vi "函数类型2测试.vi"() -> ()   [LabVIEW 2010]
uses:
  全局量/试验配置信息.vi
panel:
  out "starttest":bool
  in  "记录跳变次数":i32
  in  "变化量":dbl
  in  "当前波动值":dbl
  in  "最近一次跳变防线值":i32
  out "bRecv":bool
  out "bSend":bool
  in  "发送值状态":i32
  in  "反馈值":i32
  in  "发送值":dbl
  out "合格？":bool[][](array[boolean])
  in  "btn_反选":bool
  in  "btn_全选":bool
  out "退出？":bool
  in  "数组_选择":bool[](array[boolean])
  in  "第几组数据":i32
  in  "A_32":bool
  in  "A_31":bool
  in  "A_30":bool
  in  "A_29":bool
  in  "A_28":bool
  in  "A_27":bool
  in  "A_26":bool
  in  "A_25":bool
  in  "A_24":bool
  in  "A_23":bool
  in  "A_22":bool
  in  "A_21":bool
  in  "A_20":bool
  in  "A_19":bool
  in  "A_18":bool
  in  "A_17":bool
  in  "A_16":bool
  in  "A_15":bool
  in  "A_14":bool
  in  "A_13":bool
  in  "A_12":bool
  in  "A_11":bool
  in  "A_10":bool
  in  "A_9":bool
  in  "A_8":bool
  in  "A_7":bool
  in  "A_6":bool
  in  "A_5":bool
  in  "A_4":bool
  in  "A_3":bool
  in  "A_2":bool
  in  "A_1":bool
  in  "btn_取消":bool
  in  "btn_开始测试":bool
  out "light_32":bool
  out "light_31":bool
  out "light_30":bool
  out "light_29":bool
  out "light_28":bool
  out "light_27":bool
  out "light_26":bool
  out "light_25":bool
  out "light_24":bool
  out "light_23":bool
  out "light_22":bool
  out "light_21":bool
  out "light_20":bool
  out "light_19":bool
  out "light_18":bool
  out "light_17":bool
  out "light_16":bool
  out "light_15":bool
  out "light_14":bool
  out "light_13":bool
  out "light_12":bool
  out "light_11":bool
  out "light_10":bool
  out "light_9":bool
  out "light_8":bool
  out "light_7":bool
  out "light_6":bool
  out "light_5":bool
  out "light_4":bool
  out "light_3":bool
  out "light_2":bool
  out "light_1":bool
  in  "跳变值 2":dbl[](array[numeric])
  in  "跳变值 1":dbl[](array[numeric])
  out "Analog_back":string[][](table) caption="表格"
  in  "Analog_IN":string[][](table) caption="表格"
  # "反馈电平状态"
  # "模拟量输入值（V）"
  # "SEND_RISE = 1,//递增\n\tSEND_SUB = 2,//递减\n\tSEND_OVER = 3//发送完毕"
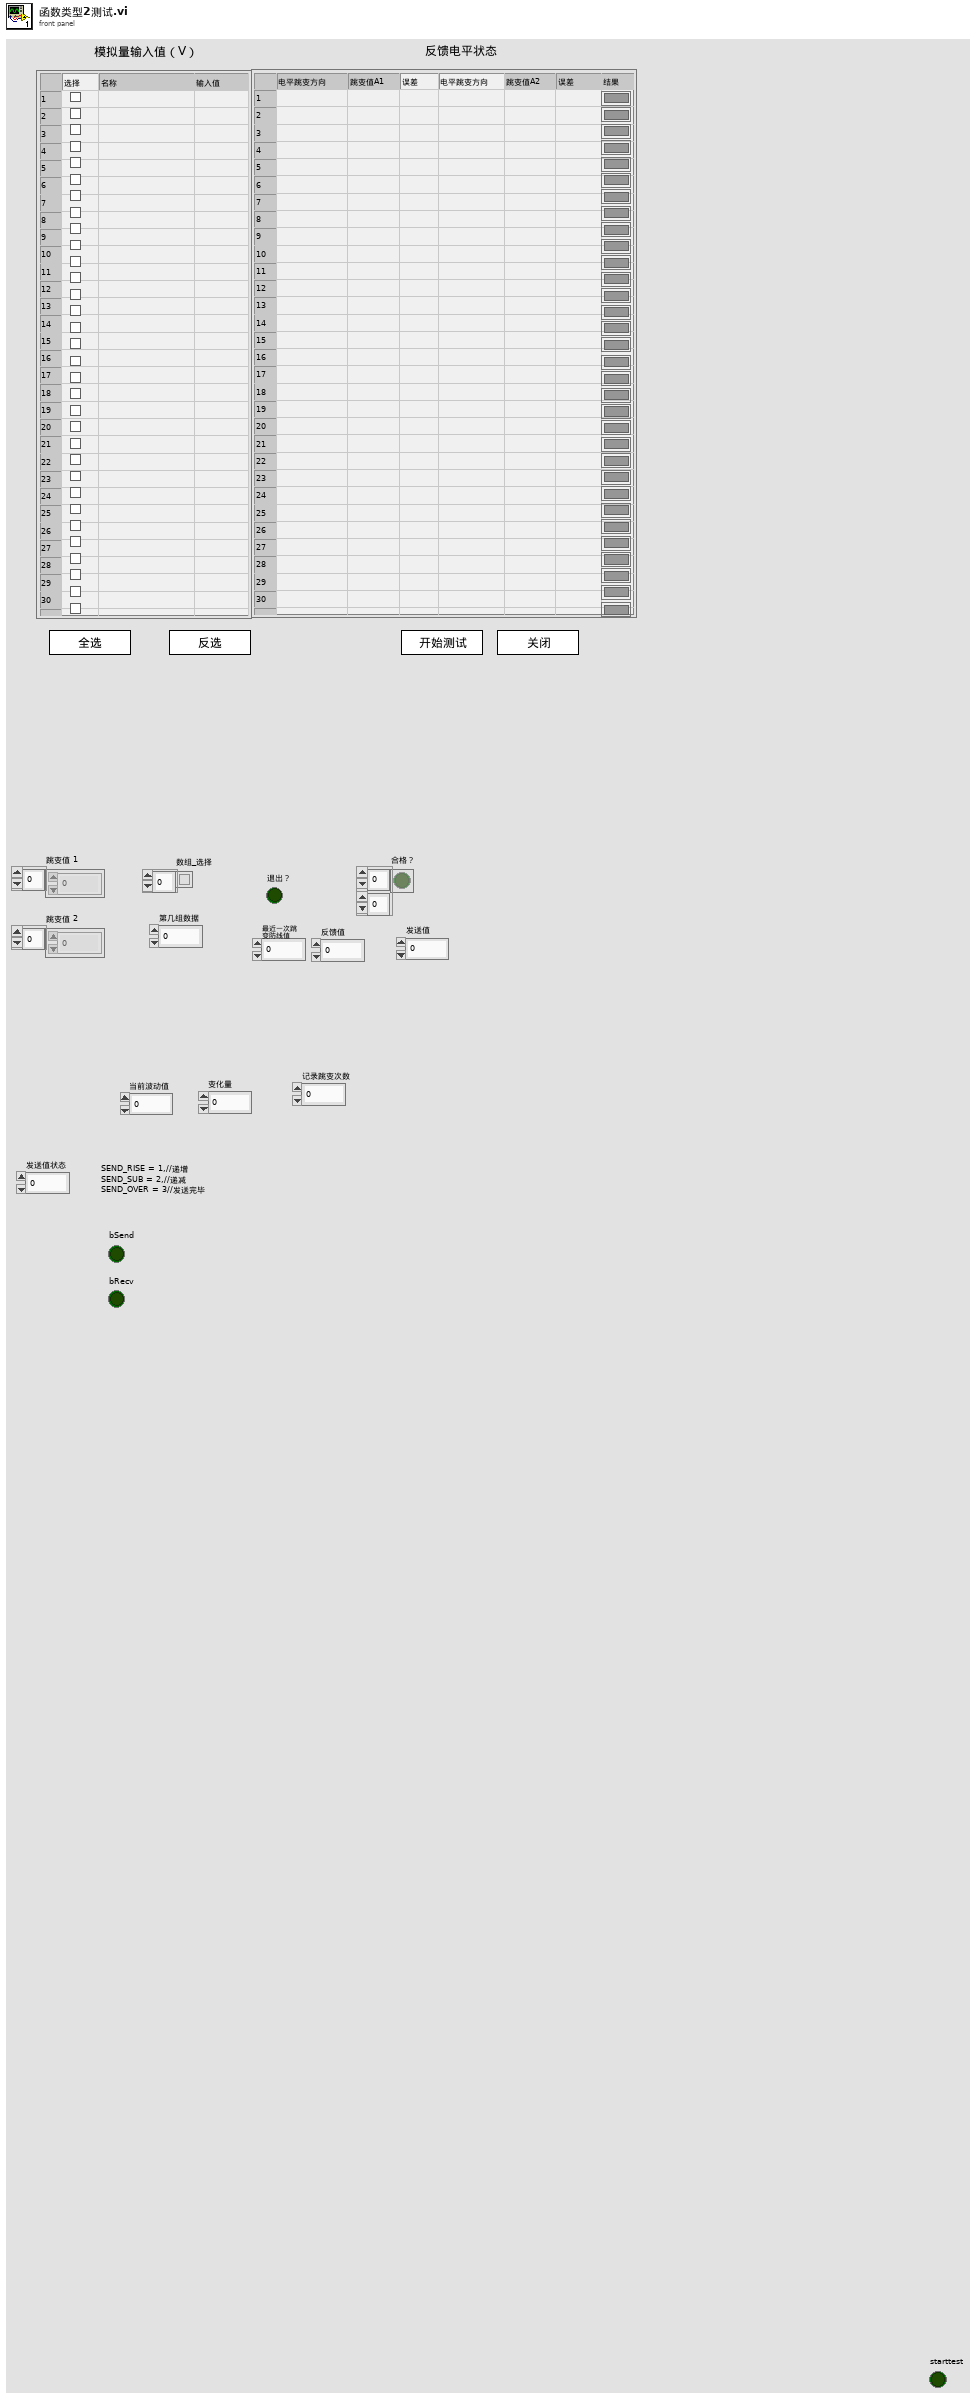
[diagram p1: front panel]
types:
  T1 = enum8{"Enabled", "Disabled", "Disabled and Grayed Out"}
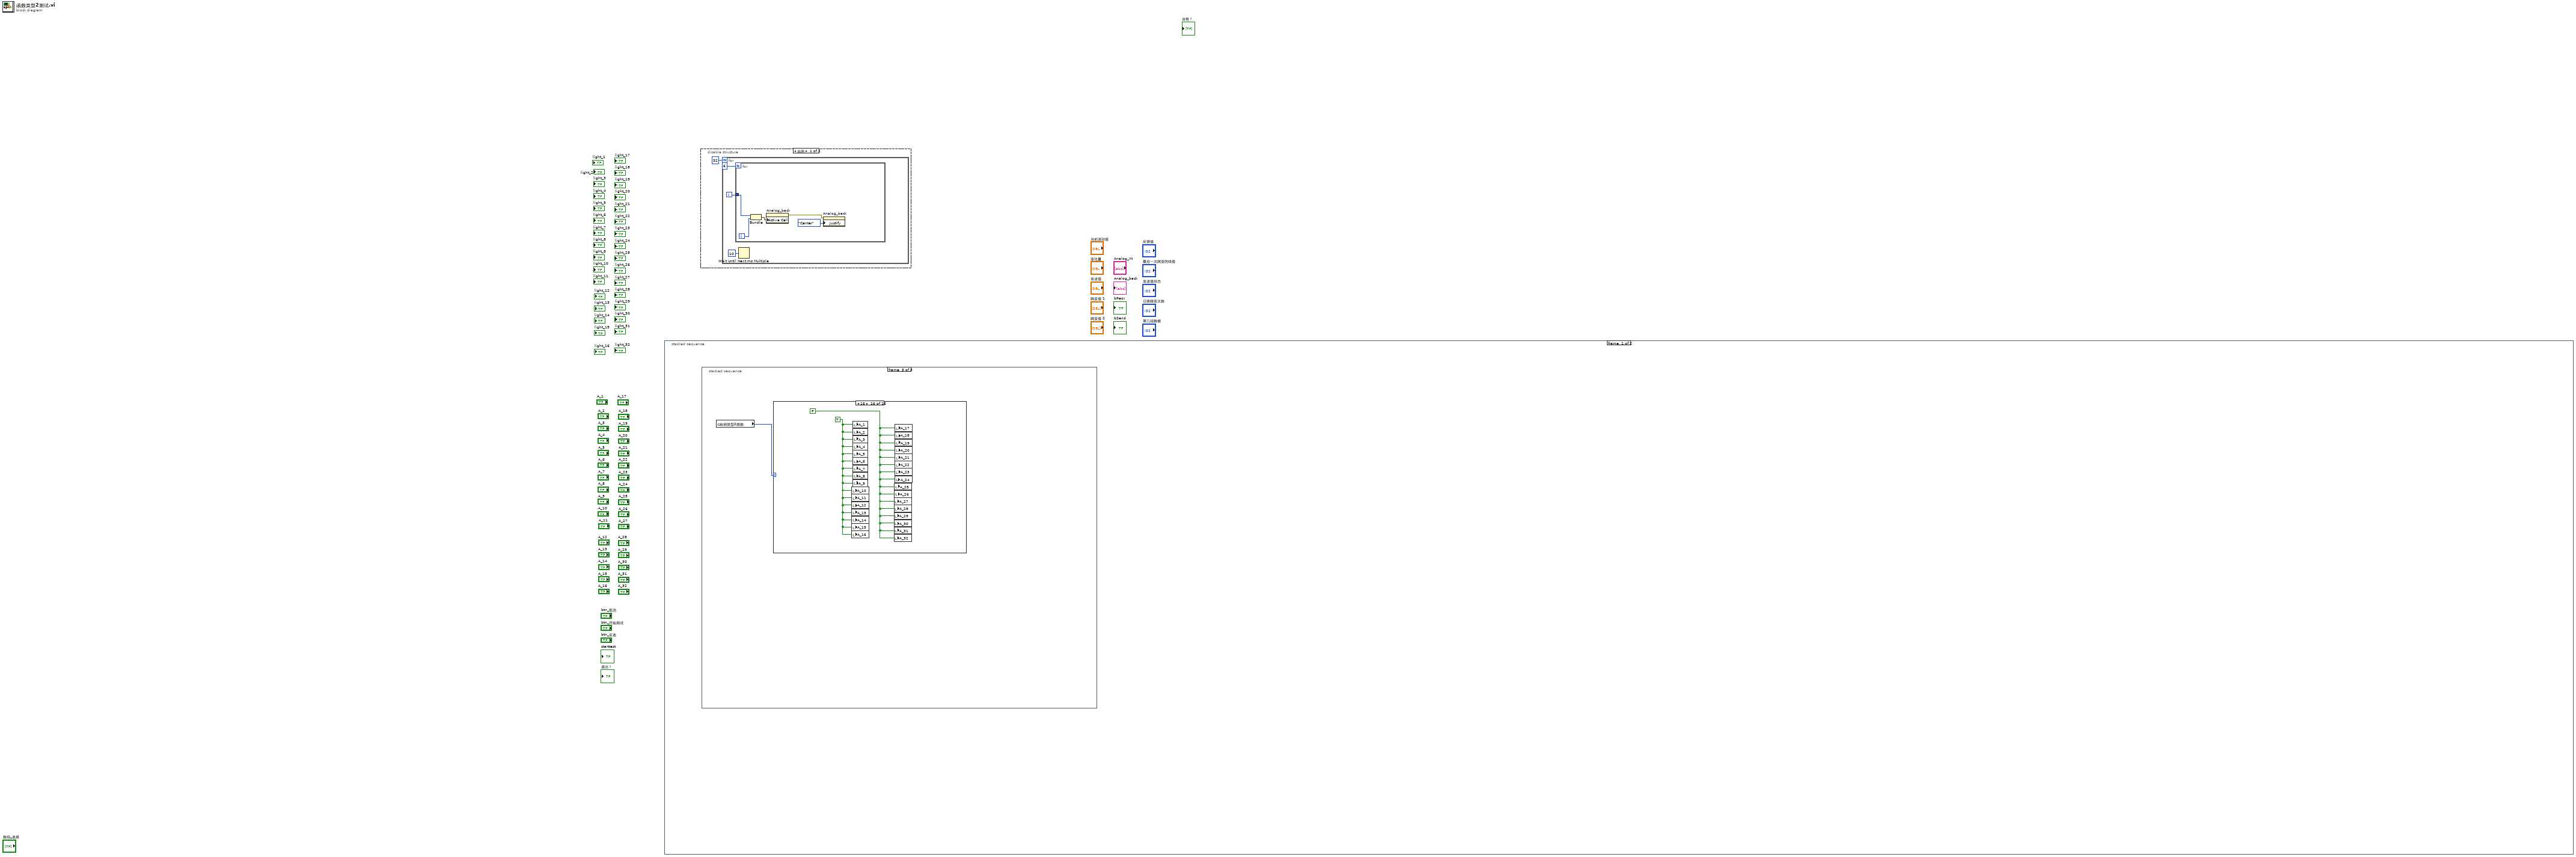
[diagram p0: block diagram]
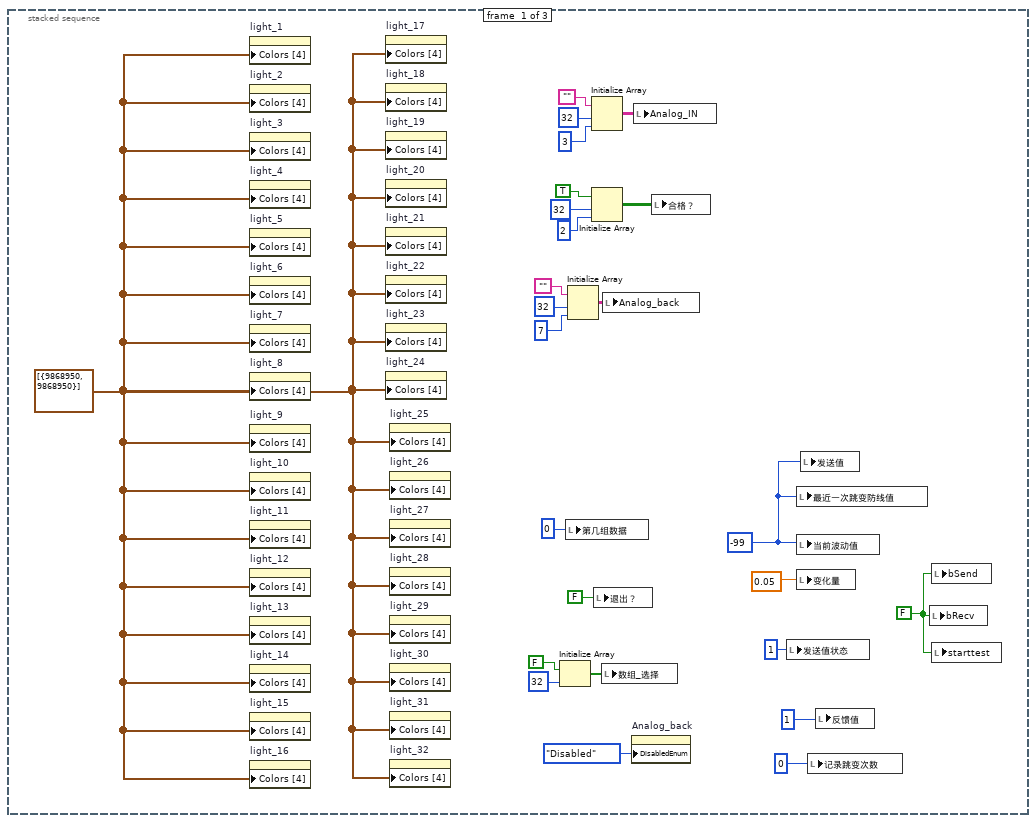
[diagram p3: hidden frame]
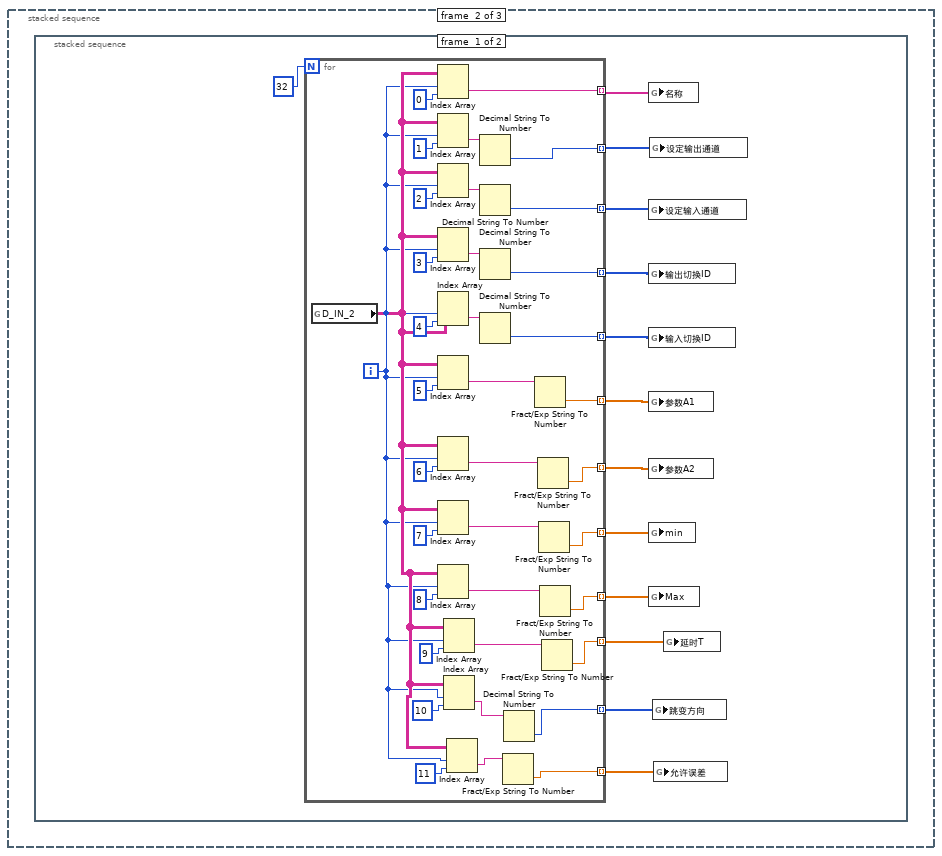
[diagram p4: hidden frame]
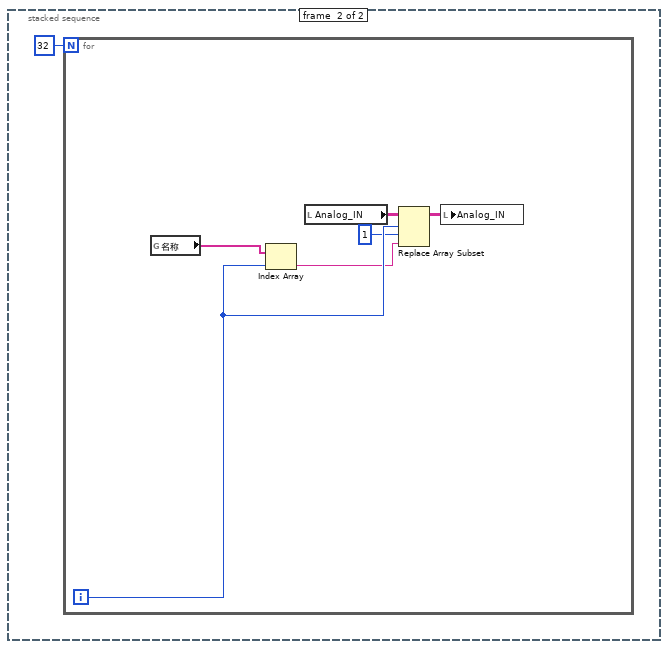
[diagram p5: hidden frame]
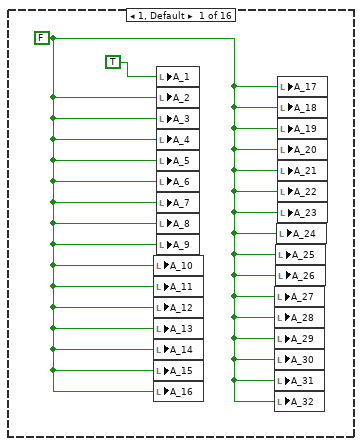
[diagram p6: hidden frame]
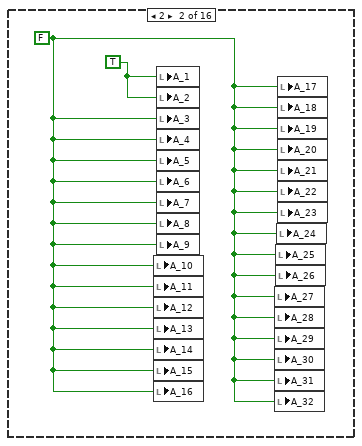
[diagram p7: hidden frame]
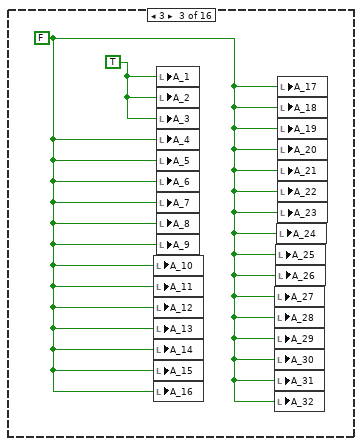
[diagram p8: hidden frame]
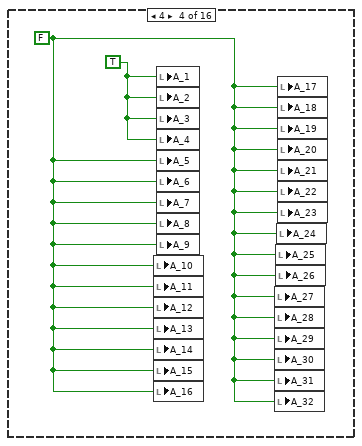
[diagram p9: hidden frame]
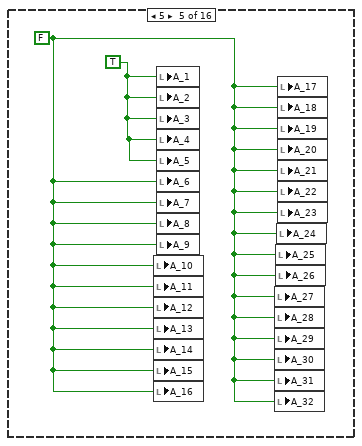
[diagram p10: hidden frame]
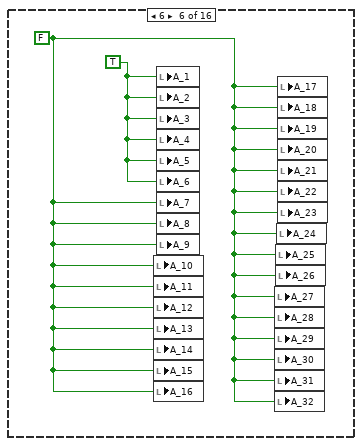
[diagram p11: hidden frame]
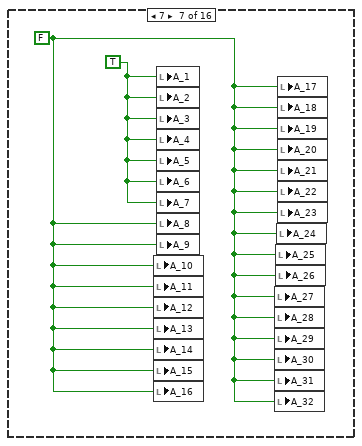
[diagram p12: hidden frame]
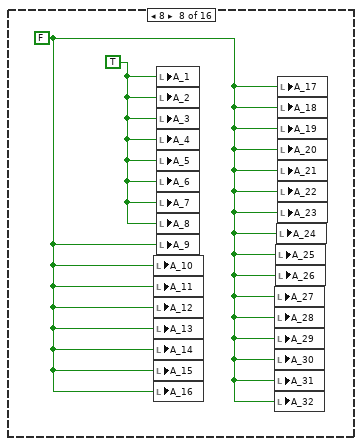
[diagram p13: hidden frame]
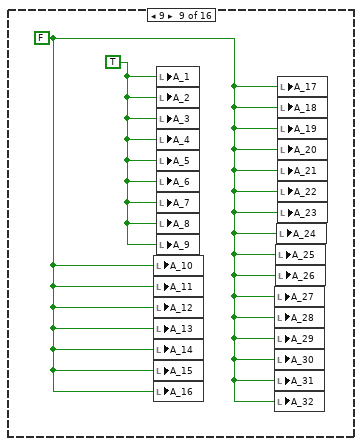
[diagram p14: hidden frame]
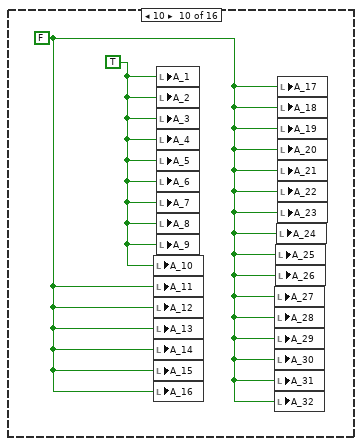
[diagram p15: hidden frame]
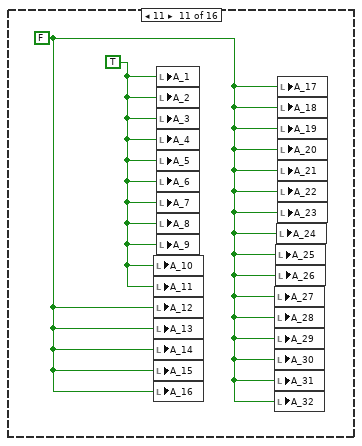
[diagram p16: hidden frame]
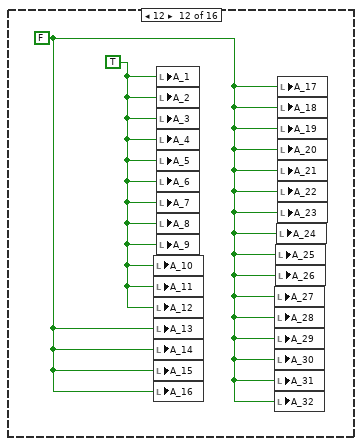
[diagram p17: hidden frame]
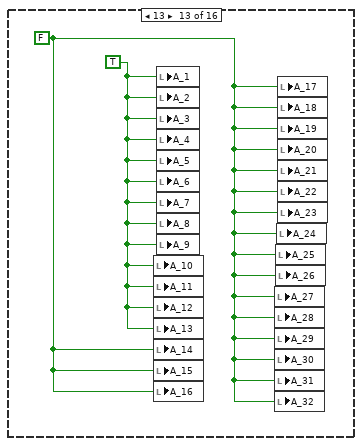
[diagram p18: hidden frame]
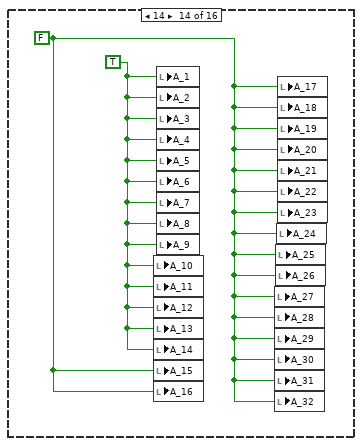
[diagram p19: hidden frame]
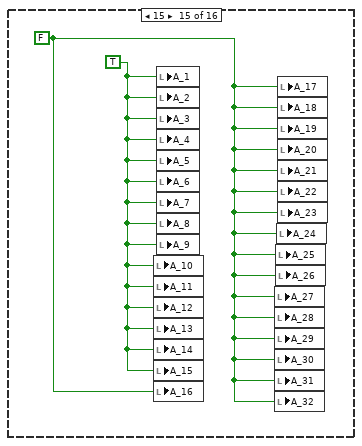
[diagram p20: hidden frame]
diagram:
  n1 = stacked-sequence {
    frame #0 {
      n2 = stacked-sequence {
        frame #0 {
          w9 = -99
          w6 = FALSE
          w21 = cluster{u32, u32}[] [{9868950, 9868950}]
          n3 = property on="light_1" class="Bool (严格)"("Colors [4]"=w21) -> ()  [unwired: 2 in, 2 out]
          n4 = property on="light_2" class="Bool (严格)"("Colors [4]"=w21) -> ()  [unwired: 2 in, 2 out]
          n5 = property on="light_3" class="Bool (严格)"("Colors [4]"=w21) -> ()  [unwired: 2 in, 2 out]
          n6 = property on="light_4" class="Bool (严格)"("Colors [4]"=w21) -> ()  [unwired: 2 in, 2 out]
          n7 = property on="light_5" class="Bool (严格)"("Colors [4]"=w21) -> ()  [unwired: 2 in, 2 out]
          n8 = property on="light_6" class="Bool (严格)"("Colors [4]"=w21) -> ()  [unwired: 2 in, 2 out]
          n9 = property on="light_7" class="Bool (严格)"("Colors [4]"=w21) -> ()  [unwired: 2 in, 2 out]
          n10 = property on="light_8" class="Bool (严格)"("Colors [4]"=w21) -> ()  [unwired: 2 in, 2 out]
          n11 = property on="light_9" class="Bool (严格)"("Colors [4]"=w21) -> ()  [unwired: 2 in, 2 out]
          n12 = property on="light_10" class="Bool (严格)"("Colors [4]"=w21) -> ()  [unwired: 2 in, 2 out]
          n13 = property on="light_11" class="Bool (严格)"("Colors [4]"=w21) -> ()  [unwired: 2 in, 2 out]
          n14 = property on="light_12" class="Bool (严格)"("Colors [4]"=w21) -> ()  [unwired: 2 in, 2 out]
          n15 = property on="light_13" class="Bool (严格)"("Colors [4]"=w21) -> ()  [unwired: 2 in, 2 out]
          n16 = property on="light_14" class="Bool (严格)"("Colors [4]"=w21) -> ()  [unwired: 2 in, 2 out]
          n17 = property on="light_15" class="Bool (严格)"("Colors [4]"=w21) -> ()  [unwired: 2 in, 2 out]
          n18 = property on="light_16" class="Bool (严格)"("Colors [4]"=w21) -> ()  [unwired: 2 in, 2 out]
          n19 = property on="light_17" class="Bool (严格)"("Colors [4]"=w21) -> ()  [unwired: 2 in, 2 out]
          n20 = property on="light_18" class="Bool (严格)"("Colors [4]"=w21) -> ()  [unwired: 2 in, 2 out]
          n21 = property on="light_19" class="Bool (严格)"("Colors [4]"=w21) -> ()  [unwired: 2 in, 2 out]
          n22 = property on="light_20" class="Bool (严格)"("Colors [4]"=w21) -> ()  [unwired: 2 in, 2 out]
          n23 = property on="light_21" class="Bool (严格)"("Colors [4]"=w21) -> ()  [unwired: 2 in, 2 out]
          n24 = property on="light_22" class="Bool (严格)"("Colors [4]"=w21) -> ()  [unwired: 2 in, 2 out]
          n25 = property on="light_23" class="Bool (严格)"("Colors [4]"=w21) -> ()  [unwired: 2 in, 2 out]
          n26 = property on="light_24" class="Bool (严格)"("Colors [4]"=w21) -> ()  [unwired: 2 in, 2 out]
          n27 = property on="light_25" class="Bool (严格)"("Colors [4]"=w21) -> ()  [unwired: 2 in, 2 out]
          n28 = property on="light_26" class="Bool (严格)"("Colors [4]"=w21) -> ()  [unwired: 2 in, 2 out]
          n29 = property on="light_27" class="Bool (严格)"("Colors [4]"=w21) -> ()  [unwired: 2 in, 2 out]
          n30 = property on="light_28" class="Bool (严格)"("Colors [4]"=w21) -> ()  [unwired: 2 in, 2 out]
          n31 = property on="light_29" class="Bool (严格)"("Colors [4]"=w21) -> ()  [unwired: 2 in, 2 out]
          n32 = property on="light_30" class="Bool (严格)"("Colors [4]"=w21) -> ()  [unwired: 2 in, 2 out]
          n33 = property on="light_31" class="Bool (严格)"("Colors [4]"=w21) -> ()  [unwired: 2 in, 2 out]
          n34 = property on="light_32" class="Bool (严格)"("Colors [4]"=w21) -> ()  [unwired: 2 in, 2 out]
          n35 = Initialize Array(FALSE, 32 ("维数大小")) -> (w19:bool[])
          n36 = local write "第几组数据"(0 ("第几组数据")) -> ()
          n37 = Initialize Array("", 32 ("维数大小"), 7 ("维数大小")) -> (w5:string[][])
          n38 = Initialize Array("", 32 ("维数大小"), 3 ("维数大小")) -> (w22:string[][])
          n39 = Initialize Array(TRUE, 32 ("维数大小"), 2 ("维数大小")) -> (w14:bool[][])
          n40 = local write "退出？"(FALSE ("退出？")) -> ()
          n41 = local write "数组_选择"(w19) -> ()
          n42 = local write "Analog_back"(w5) -> ()
          n43 = property on="Analog_back" class="Tbl (严格)"("DisabledEnum"=T1."Disabled" ("禁用")) -> ()  [unwired: 2 in, 2 out]
          n44 = local write "Analog_IN"(w22) -> ()
          n45 = local write "合格？"(w14) -> ()
          n46 = local write "发送值状态"(1 ("发送值状态")) -> ()
          n47 = local write "最近一次跳变防线值"(w9) -> ()
          n48 = local write "当前波动值"(w9) -> ()
          n49 = local write "变化量"(0.05) -> ()
          n50 = local write "发送值"(w9) -> ()
          n51 = local write "记录跳变次数"(0) -> ()
          n52 = local write "反馈值"(1) -> ()
          n53 = local write "bRecv"(w6) -> ()
          n54 = local write "bSend"(w6) -> ()
          n55 = local write "starttest"(w6) -> ()
        }
        frame #1 {
          n56 = stacked-sequence {
            frame #0 {
              n57 = for {
                N: 32 ("维数大小") -> [_]
                tunnel: [w74] -> w32 mode=indexing
                tunnel: [w70] -> w31 mode=indexing
                tunnel: [w68] -> w30 mode=indexing
                tunnel: [w65] -> w29 mode=indexing
                tunnel: [w62] -> w28 mode=indexing
                tunnel: [w59] -> w34 mode=indexing
                tunnel: [w56] -> w35 mode=indexing
                tunnel: [w53] -> w36 mode=indexing
                tunnel: [w50] -> w37 mode=indexing
                tunnel: [w47] -> w38 mode=indexing
                tunnel: [w40] -> w27 mode=indexing
                tunnel: [w39] -> w26 mode=indexing
                i -> [w41]
                n58 = global read "试验配置信息.vi" "D_IN_2"() -> (w42:string[][])
                n59 = Index Array(array=w42, index (row)=w41, index (col)=0 ("禁用的索引 (列)")) -> (element=w74:string)
                n60 = Index Array(array=w42, index (row)=w41, index (col)=1 ("禁用的索引 (列)")) -> (element=w67:string)
                n61 = Index Array(array=w42, index (row)=w41, index (col)=2 ("禁用的索引 (列)")) -> (element=w64:string)
                n62 = Index Array(array=w42, index (row)=w41, index (col)=3 ("禁用的索引 (列)")) -> (element=w60:string)
                n63 = Index Array(array=w42, index (row)=w41, index (col)=4 ("禁用的索引 (列)")) -> (element=w58:string)
                n64 = Index Array(array=w42, index (row)=w41, index (col)=5 ("禁用的索引 (列)")) -> (element=w55:string)
                n65 = Index Array(array=w42, index (row)=w41, index (col)=6 ("禁用的索引 (列)")) -> (element=w51:string)
                n66 = Index Array(array=w42, index (row)=w41, index (col)=7 ("禁用的索引 (列)")) -> (element=w71:string)
                n67 = Index Array(array=w42, index (row)=w41, index (col)=8 ("禁用的索引 (列)")) -> (element=w69:string)
                n68 = Index Array(array=w42, index (row)=w41, index (col)=9 ("禁用的索引 (列)")) -> (element=w48:string)
                n69 = Index Array(array=w42, index (row)=w41, index (col)=10 ("禁用的索引 (列)")) -> (element=w43:string)
                n70 = Index Array(array=w42, index (row)=w41, index (col)=11 ("禁用的索引 (列)")) -> (element=w44:string)
                n71 = Decimal String To Number(string=w67) -> (number=w65:i32)  [unwired: 2 in, 1 out]
                n72 = Decimal String To Number(string=w64) -> (number=w62:i32)  [unwired: 2 in, 1 out]
                n73 = Decimal String To Number(string=w60) -> (number=w59:i32)  [unwired: 2 in, 1 out]
                n74 = Decimal String To Number(string=w58) -> (number=w56:i32)  [unwired: 2 in, 1 out]
                n75 = Fract/Exp String To Number(string=w44) -> (number=w39:dbl)  [unwired: 3 in, 1 out]
                n76 = Decimal String To Number(string=w43) -> (number=w40:i32)  [unwired: 2 in, 1 out]
                n77 = Fract/Exp String To Number(string=w55) -> (number=w53:dbl)  [unwired: 3 in, 1 out]
                n78 = Fract/Exp String To Number(string=w51) -> (number=w50:dbl)  [unwired: 3 in, 1 out]
                n79 = Fract/Exp String To Number(string=w71) -> (number=w70:dbl)  [unwired: 3 in, 1 out]
                n80 = Fract/Exp String To Number(string=w69) -> (number=w68:dbl)  [unwired: 3 in, 1 out]
                n81 = Fract/Exp String To Number(string=w48) -> (number=w47:dbl)  [unwired: 3 in, 1 out]
              }
              n82 = global write "试验配置信息.vi" "名称"(w32) -> ()
              n83 = global write "试验配置信息.vi" "设定输入通道"(w28) -> ()
              n84 = global write "试验配置信息.vi" "输出切换ID"(w34) -> ()
              n85 = global write "试验配置信息.vi" "输入切换ID"(w35) -> ()
              n86 = global write "试验配置信息.vi" "参数A1"(w36) -> ()
              n87 = global write "试验配置信息.vi" "参数A2"(w37) -> ()
              n88 = global write "试验配置信息.vi" "min"(w31) -> ()
              n89 = global write "试验配置信息.vi" "Max"(w30) -> ()
              n90 = global write "试验配置信息.vi" "设定输出通道"(w29) -> ()
              n91 = global write "试验配置信息.vi" "跳变方向"(w27) -> ()
              n92 = global write "试验配置信息.vi" "允许误差"(w26) -> ()
              n93 = global write "试验配置信息.vi" "延时T"(w38) -> ()
            }
            frame #1 {
              n94 = for {
                N: 32 -> [_]
                i -> [w79]
                n95 = global read "试验配置信息.vi" "名称"() -> (w82:string[])
                n96 = Index Array(array=w82, index=w79) -> (element=w78:string)
                n97 = local read "Analog_IN"() -> (w81:string[][])
                n98 = Replace Array Subset(array=w81, new element=w78, index (row)=w79, index (col)=1 ("禁用的索引 (列)")) -> (w80:string[][])
                n99 = local write "Analog_IN"(w80) -> ()
              }
            }
          }
        }
        frame #2 {
          n100 = global read "试验配置信息.vi" "自测类型2路数"() -> (w83:i32)
          n101 = case shown="16" w83 {
            frame 1, Default {
              w85 = FALSE
              n102 = local write "A_10"(w85) -> ()
              n103 = local write "A_11"(w85) -> ()
              n104 = local write "A_12"(w85) -> ()
              n105 = local write "A_13"(w85) -> ()
              n106 = local write "A_14"(w85) -> ()
              n107 = local write "A_15"(w85) -> ()
              n108 = local write "A_16"(w85) -> ()
              n109 = local write "A_1"(TRUE) -> ()
              n110 = local write "A_2"(w85) -> ()
              n111 = local write "A_3"(w85) -> ()
              n112 = local write "A_4"(w85) -> ()
              n113 = local write "A_5"(w85) -> ()
              n114 = local write "A_6"(w85) -> ()
              n115 = local write "A_7"(w85) -> ()
              n116 = local write "A_8"(w85) -> ()
              n117 = local write "A_9"(w85) -> ()
              n118 = local write "A_27"(w85) -> ()
              n119 = local write "A_28"(w85) -> ()
              n120 = local write "A_29"(w85) -> ()
              n121 = local write "A_30"(w85) -> ()
              n122 = local write "A_31"(w85) -> ()
              n123 = local write "A_32"(w85) -> ()
              n124 = local write "A_25"(w85) -> ()
              n125 = local write "A_26"(w85) -> ()
              n126 = local write "A_24"(w85) -> ()
              n127 = local write "A_17"(w85) -> ()
              n128 = local write "A_18"(w85) -> ()
              n129 = local write "A_19"(w85) -> ()
              n130 = local write "A_20"(w85) -> ()
              n131 = local write "A_21"(w85) -> ()
              n132 = local write "A_22"(w85) -> ()
              n133 = local write "A_23"(w85) -> ()
            }
            frame 2 {
              w86 = TRUE
              w87 = FALSE
              n134 = local write "A_10"(w87) -> ()
              n135 = local write "A_11"(w87) -> ()
              n136 = local write "A_12"(w87) -> ()
              n137 = local write "A_13"(w87) -> ()
              n138 = local write "A_14"(w87) -> ()
              n139 = local write "A_15"(w87) -> ()
              n140 = local write "A_16"(w87) -> ()
              n141 = local write "A_1"(w86) -> ()
              n142 = local write "A_2"(w86) -> ()
              n143 = local write "A_3"(w87) -> ()
              n144 = local write "A_4"(w87) -> ()
              n145 = local write "A_5"(w87) -> ()
              n146 = local write "A_6"(w87) -> ()
              n147 = local write "A_7"(w87) -> ()
              n148 = local write "A_8"(w87) -> ()
              n149 = local write "A_9"(w87) -> ()
              n150 = local write "A_27"(w87) -> ()
              n151 = local write "A_28"(w87) -> ()
              n152 = local write "A_29"(w87) -> ()
              n153 = local write "A_30"(w87) -> ()
              n154 = local write "A_31"(w87) -> ()
              n155 = local write "A_32"(w87) -> ()
              n156 = local write "A_25"(w87) -> ()
              n157 = local write "A_26"(w87) -> ()
              n158 = local write "A_24"(w87) -> ()
              n159 = local write "A_17"(w87) -> ()
              n160 = local write "A_18"(w87) -> ()
              n161 = local write "A_19"(w87) -> ()
              n162 = local write "A_20"(w87) -> ()
              n163 = local write "A_21"(w87) -> ()
              n164 = local write "A_22"(w87) -> ()
              n165 = local write "A_23"(w87) -> ()
            }
            frame 3 {
              w88 = TRUE
              w89 = FALSE
              n166 = local write "A_10"(w89) -> ()
              n167 = local write "A_11"(w89) -> ()
              n168 = local write "A_12"(w89) -> ()
              n169 = local write "A_13"(w89) -> ()
              n170 = local write "A_14"(w89) -> ()
              n171 = local write "A_15"(w89) -> ()
              n172 = local write "A_16"(w89) -> ()
              n173 = local write "A_1"(w88) -> ()
              n174 = local write "A_2"(w88) -> ()
              n175 = local write "A_3"(w88) -> ()
              n176 = local write "A_4"(w89) -> ()
              n177 = local write "A_5"(w89) -> ()
              n178 = local write "A_6"(w89) -> ()
              n179 = local write "A_7"(w89) -> ()
              n180 = local write "A_8"(w89) -> ()
              n181 = local write "A_9"(w89) -> ()
              n182 = local write "A_27"(w89) -> ()
              n183 = local write "A_28"(w89) -> ()
              n184 = local write "A_29"(w89) -> ()
              n185 = local write "A_30"(w89) -> ()
              n186 = local write "A_31"(w89) -> ()
              n187 = local write "A_32"(w89) -> ()
              n188 = local write "A_25"(w89) -> ()
              n189 = local write "A_26"(w89) -> ()
              n190 = local write "A_24"(w89) -> ()
              n191 = local write "A_17"(w89) -> ()
              n192 = local write "A_18"(w89) -> ()
              n193 = local write "A_19"(w89) -> ()
              n194 = local write "A_20"(w89) -> ()
              n195 = local write "A_21"(w89) -> ()
              n196 = local write "A_22"(w89) -> ()
              n197 = local write "A_23"(w89) -> ()
            }
            frame 4 {
              w90 = TRUE
              w91 = FALSE
              n198 = local write "A_10"(w91) -> ()
              n199 = local write "A_11"(w91) -> ()
              n200 = local write "A_12"(w91) -> ()
              n201 = local write "A_13"(w91) -> ()
              n202 = local write "A_14"(w91) -> ()
              n203 = local write "A_15"(w91) -> ()
              n204 = local write "A_16"(w91) -> ()
              n205 = local write "A_1"(w90) -> ()
              n206 = local write "A_2"(w90) -> ()
              n207 = local write "A_3"(w90) -> ()
              n208 = local write "A_4"(w90) -> ()
              n209 = local write "A_5"(w91) -> ()
              n210 = local write "A_6"(w91) -> ()
              n211 = local write "A_7"(w91) -> ()
              n212 = local write "A_8"(w91) -> ()
              n213 = local write "A_9"(w91) -> ()
              n214 = local write "A_27"(w91) -> ()
              n215 = local write "A_28"(w91) -> ()
              n216 = local write "A_29"(w91) -> ()
              n217 = local write "A_30"(w91) -> ()
              n218 = local write "A_31"(w91) -> ()
              n219 = local write "A_32"(w91) -> ()
              n220 = local write "A_25"(w91) -> ()
              n221 = local write "A_26"(w91) -> ()
              n222 = local write "A_24"(w91) -> ()
              n223 = local write "A_17"(w91) -> ()
              n224 = local write "A_18"(w91) -> ()
              n225 = local write "A_19"(w91) -> ()
              n226 = local write "A_20"(w91) -> ()
              n227 = local write "A_21"(w91) -> ()
              n228 = local write "A_22"(w91) -> ()
              n229 = local write "A_23"(w91) -> ()
            }
            frame 5 {
              w92 = TRUE
              w93 = FALSE
              n230 = local write "A_10"(w93) -> ()
              n231 = local write "A_11"(w93) -> ()
              n232 = local write "A_12"(w93) -> ()
              n233 = local write "A_13"(w93) -> ()
              n234 = local write "A_14"(w93) -> ()
              n235 = local write "A_15"(w93) -> ()
              n236 = local write "A_16"(w93) -> ()
              n237 = local write "A_1"(w92) -> ()
              n238 = local write "A_2"(w92) -> ()
              n239 = local write "A_3"(w92) -> ()
              n240 = local write "A_4"(w92) -> ()
              n241 = local write "A_5"(w92) -> ()
              n242 = local write "A_6"(w93) -> ()
              n243 = local write "A_7"(w93) -> ()
              n244 = local write "A_8"(w93) -> ()
              n245 = local write "A_9"(w93) -> ()
              n246 = local write "A_27"(w93) -> ()
              n247 = local write "A_28"(w93) -> ()
              n248 = local write "A_29"(w93) -> ()
              n249 = local write "A_30"(w93) -> ()
              n250 = local write "A_31"(w93) -> ()
              n251 = local write "A_32"(w93) -> ()
              n252 = local write "A_25"(w93) -> ()
              n253 = local write "A_26"(w93) -> ()
              n254 = local write "A_24"(w93) -> ()
              n255 = local write "A_17"(w93) -> ()
              n256 = local write "A_18"(w93) -> ()
              n257 = local write "A_19"(w93) -> ()
              n258 = local write "A_20"(w93) -> ()
              n259 = local write "A_21"(w93) -> ()
              n260 = local write "A_22"(w93) -> ()
              n261 = local write "A_23"(w93) -> ()
            }
            frame 6 {
              w94 = TRUE
              w95 = FALSE
              n262 = local write "A_10"(w95) -> ()
              n263 = local write "A_11"(w95) -> ()
              n264 = local write "A_12"(w95) -> ()
              n265 = local write "A_13"(w95) -> ()
              n266 = local write "A_14"(w95) -> ()
              n267 = local write "A_15"(w95) -> ()
              n268 = local write "A_16"(w95) -> ()
              n269 = local write "A_1"(w94) -> ()
              n270 = local write "A_2"(w94) -> ()
              n271 = local write "A_3"(w94) -> ()
              n272 = local write "A_4"(w94) -> ()
              n273 = local write "A_5"(w94) -> ()
              n274 = local write "A_6"(w94) -> ()
              n275 = local write "A_7"(w95) -> ()
              n276 = local write "A_8"(w95) -> ()
              n277 = local write "A_9"(w95) -> ()
              n278 = local write "A_27"(w95) -> ()
              n279 = local write "A_28"(w95) -> ()
              n280 = local write "A_29"(w95) -> ()
              n281 = local write "A_30"(w95) -> ()
              n282 = local write "A_31"(w95) -> ()
              n283 = local write "A_32"(w95) -> ()
              n284 = local write "A_25"(w95) -> ()
              n285 = local write "A_26"(w95) -> ()
              n286 = local write "A_24"(w95) -> ()
              n287 = local write "A_17"(w95) -> ()
              n288 = local write "A_18"(w95) -> ()
              n289 = local write "A_19"(w95) -> ()
              n290 = local write "A_20"(w95) -> ()
              n291 = local write "A_21"(w95) -> ()
              n292 = local write "A_22"(w95) -> ()
              n293 = local write "A_23"(w95) -> ()
            }
            frame 7 {
              w96 = TRUE
              w97 = FALSE
              n294 = local write "A_10"(w97) -> ()
              n295 = local write "A_11"(w97) -> ()
              n296 = local write "A_12"(w97) -> ()
              n297 = local write "A_13"(w97) -> ()
              n298 = local write "A_14"(w97) -> ()
              n299 = local write "A_15"(w97) -> ()
              n300 = local write "A_16"(w97) -> ()
              n301 = local write "A_1"(w96) -> ()
              n302 = local write "A_2"(w96) -> ()
              n303 = local write "A_3"(w96) -> ()
              n304 = local write "A_4"(w96) -> ()
              n305 = local write "A_5"(w96) -> ()
              n306 = local write "A_6"(w96) -> ()
              n307 = local write "A_7"(w96) -> ()
              n308 = local write "A_8"(w97) -> ()
              n309 = local write "A_9"(w97) -> ()
              n310 = local write "A_27"(w97) -> ()
              n311 = local write "A_28"(w97) -> ()
              n312 = local write "A_29"(w97) -> ()
              n313 = local write "A_30"(w97) -> ()
              n314 = local write "A_31"(w97) -> ()
              n315 = local write "A_32"(w97) -> ()
              n316 = local write "A_25"(w97) -> ()
              n317 = local write "A_26"(w97) -> ()
              n318 = local write "A_24"(w97) -> ()
              n319 = local write "A_17"(w97) -> ()
              n320 = local write "A_18"(w97) -> ()
              n321 = local write "A_19"(w97) -> ()
              n322 = local write "A_20"(w97) -> ()
              n323 = local write "A_21"(w97) -> ()
              n324 = local write "A_22"(w97) -> ()
              n325 = local write "A_23"(w97) -> ()
            }
            frame 8 {
              w98 = TRUE
              w99 = FALSE
              n326 = local write "A_10"(w99) -> ()
              n327 = local write "A_11"(w99) -> ()
              n328 = local write "A_12"(w99) -> ()
              n329 = local write "A_13"(w99) -> ()
              n330 = local write "A_14"(w99) -> ()
              n331 = local write "A_15"(w99) -> ()
              n332 = local write "A_16"(w99) -> ()
              n333 = local write "A_1"(w98) -> ()
              n334 = local write "A_2"(w98) -> ()
              n335 = local write "A_3"(w98) -> ()
              n336 = local write "A_4"(w98) -> ()
              n337 = local write "A_5"(w98) -> ()
              n338 = local write "A_6"(w98) -> ()
              n339 = local write "A_7"(w98) -> ()
              n340 = local write "A_8"(w98) -> ()
              n341 = local write "A_9"(w99) -> ()
              n342 = local write "A_27"(w99) -> ()
              n343 = local write "A_28"(w99) -> ()
              n344 = local write "A_29"(w99) -> ()
              n345 = local write "A_30"(w99) -> ()
              n346 = local write "A_31"(w99) -> ()
              n347 = local write "A_32"(w99) -> ()
              n348 = local write "A_25"(w99) -> ()
              n349 = local write "A_26"(w99) -> ()
              n350 = local write "A_24"(w99) -> ()
              n351 = local write "A_17"(w99) -> ()
              n352 = local write "A_18"(w99) -> ()
              n353 = local write "A_19"(w99) -> ()
              n354 = local write "A_20"(w99) -> ()
              n355 = local write "A_21"(w99) -> ()
              n356 = local write "A_22"(w99) -> ()
              n357 = local write "A_23"(w99) -> ()
            }
            frame 9 {
              w100 = TRUE
              w101 = FALSE
              n358 = local write "A_10"(w101) -> ()
              n359 = local write "A_11"(w101) -> ()
              n360 = local write "A_12"(w101) -> ()
              n361 = local write "A_13"(w101) -> ()
              n362 = local write "A_14"(w101) -> ()
              n363 = local write "A_15"(w101) -> ()
              n364 = local write "A_16"(w101) -> ()
              n365 = local write "A_1"(w100) -> ()
              n366 = local write "A_2"(w100) -> ()
              n367 = local write "A_3"(w100) -> ()
              n368 = local write "A_4"(w100) -> ()
              n369 = local write "A_5"(w100) -> ()
              n370 = local write "A_6"(w100) -> ()
              n371 = local write "A_7"(w100) -> ()
              n372 = local write "A_8"(w100) -> ()
              n373 = local write "A_9"(w100) -> ()
              n374 = local write "A_27"(w101) -> ()
              n375 = local write "A_28"(w101) -> ()
              n376 = local write "A_29"(w101) -> ()
              n377 = local write "A_30"(w101) -> ()
              n378 = local write "A_31"(w101) -> ()
              n379 = local write "A_32"(w101) -> ()
              n380 = local write "A_25"(w101) -> ()
              n381 = local write "A_26"(w101) -> ()
              n382 = local write "A_24"(w101) -> ()
              n383 = local write "A_17"(w101) -> ()
              n384 = local write "A_18"(w101) -> ()
              n385 = local write "A_19"(w101) -> ()
              n386 = local write "A_20"(w101) -> ()
              n387 = local write "A_21"(w101) -> ()
              n388 = local write "A_22"(w101) -> ()
              n389 = local write "A_23"(w101) -> ()
            }
            frame 10 {
              w102 = TRUE
              w103 = FALSE
              n390 = local write "A_10"(w102) -> ()
              n391 = local write "A_11"(w103) -> ()
              n392 = local write "A_12"(w103) -> ()
              n393 = local write "A_13"(w103) -> ()
              n394 = local write "A_14"(w103) -> ()
              n395 = local write "A_15"(w103) -> ()
              n396 = local write "A_16"(w103) -> ()
              n397 = local write "A_1"(w102) -> ()
              n398 = local write "A_2"(w102) -> ()
              n399 = local write "A_3"(w102) -> ()
              n400 = local write "A_4"(w102) -> ()
              n401 = local write "A_5"(w102) -> ()
              n402 = local write "A_6"(w102) -> ()
              n403 = local write "A_7"(w102) -> ()
              n404 = local write "A_8"(w102) -> ()
              n405 = local write "A_9"(w102) -> ()
              n406 = local write "A_27"(w103) -> ()
              n407 = local write "A_28"(w103) -> ()
              n408 = local write "A_29"(w103) -> ()
              n409 = local write "A_30"(w103) -> ()
              n410 = local write "A_31"(w103) -> ()
              n411 = local write "A_32"(w103) -> ()
              n412 = local write "A_25"(w103) -> ()
              n413 = local write "A_26"(w103) -> ()
              n414 = local write "A_24"(w103) -> ()
              n415 = local write "A_17"(w103) -> ()
              n416 = local write "A_18"(w103) -> ()
              n417 = local write "A_19"(w103) -> ()
              n418 = local write "A_20"(w103) -> ()
              n419 = local write "A_21"(w103) -> ()
              n420 = local write "A_22"(w103) -> ()
              n421 = local write "A_23"(w103) -> ()
            }
            frame 11 {
              w104 = TRUE
              w105 = FALSE
              n422 = local write "A_10"(w104) -> ()
              n423 = local write "A_11"(w104) -> ()
              n424 = local write "A_12"(w105) -> ()
              n425 = local write "A_13"(w105) -> ()
              n426 = local write "A_14"(w105) -> ()
              n427 = local write "A_15"(w105) -> ()
              n428 = local write "A_16"(w105) -> ()
              n429 = local write "A_1"(w104) -> ()
              n430 = local write "A_2"(w104) -> ()
              n431 = local write "A_3"(w104) -> ()
              n432 = local write "A_4"(w104) -> ()
              n433 = local write "A_5"(w104) -> ()
              n434 = local write "A_6"(w104) -> ()
              n435 = local write "A_7"(w104) -> ()
              n436 = local write "A_8"(w104) -> ()
              n437 = local write "A_9"(w104) -> ()
              n438 = local write "A_27"(w105) -> ()
              n439 = local write "A_28"(w105) -> ()
              n440 = local write "A_29"(w105) -> ()
              n441 = local write "A_30"(w105) -> ()
              n442 = local write "A_31"(w105) -> ()
              n443 = local write "A_32"(w105) -> ()
              n444 = local write "A_25"(w105) -> ()
              n445 = local write "A_26"(w105) -> ()
              n446 = local write "A_24"(w105) -> ()
              n447 = local write "A_17"(w105) -> ()
              n448 = local write "A_18"(w105) -> ()
              n449 = local write "A_19"(w105) -> ()
              n450 = local write "A_20"(w105) -> ()
              n451 = local write "A_21"(w105) -> ()
              n452 = local write "A_22"(w105) -> ()
              n453 = local write "A_23"(w105) -> ()
            }
            frame 12 {
              w106 = TRUE
              w107 = FALSE
              n454 = local write "A_10"(w106) -> ()
              n455 = local write "A_11"(w106) -> ()
              n456 = local write "A_12"(w106) -> ()
              n457 = local write "A_13"(w107) -> ()
              n458 = local write "A_14"(w107) -> ()
              n459 = local write "A_15"(w107) -> ()
              n460 = local write "A_16"(w107) -> ()
              n461 = local write "A_1"(w106) -> ()
              n462 = local write "A_2"(w106) -> ()
              n463 = local write "A_3"(w106) -> ()
              n464 = local write "A_4"(w106) -> ()
              n465 = local write "A_5"(w106) -> ()
              n466 = local write "A_6"(w106) -> ()
              n467 = local write "A_7"(w106) -> ()
              n468 = local write "A_8"(w106) -> ()
              n469 = local write "A_9"(w106) -> ()
              n470 = local write "A_27"(w107) -> ()
              n471 = local write "A_28"(w107) -> ()
              n472 = local write "A_29"(w107) -> ()
              n473 = local write "A_30"(w107) -> ()
              n474 = local write "A_31"(w107) -> ()
              n475 = local write "A_32"(w107) -> ()
              n476 = local write "A_25"(w107) -> ()
              n477 = local write "A_26"(w107) -> ()
              n478 = local write "A_24"(w107) -> ()
              n479 = local write "A_17"(w107) -> ()
              n480 = local write "A_18"(w107) -> ()
              n481 = local write "A_19"(w107) -> ()
              n482 = local write "A_20"(w107) -> ()
              n483 = local write "A_21"(w107) -> ()
              n484 = local write "A_22"(w107) -> ()
              n485 = local write "A_23"(w107) -> ()
            }
            frame 13 {
              w108 = TRUE
              w109 = FALSE
              n486 = local write "A_10"(w108) -> ()
              n487 = local write "A_11"(w108) -> ()
              n488 = local write "A_12"(w108) -> ()
              n489 = local write "A_13"(w108) -> ()
              n490 = local write "A_14"(w109) -> ()
              n491 = local write "A_15"(w109) -> ()
              n492 = local write "A_16"(w109) -> ()
              n493 = local write "A_1"(w108) -> ()
              n494 = local write "A_2"(w108) -> ()
              n495 = local write "A_3"(w108) -> ()
              n496 = local write "A_4"(w108) -> ()
              n497 = local write "A_5"(w108) -> ()
              n498 = local write "A_6"(w108) -> ()
              n499 = local write "A_7"(w108) -> ()
              n500 = local write "A_8"(w108) -> ()
              n501 = local write "A_9"(w108) -> ()
              n502 = local write "A_27"(w109) -> ()
              n503 = local write "A_28"(w109) -> ()
              n504 = local write "A_29"(w109) -> ()
              n505 = local write "A_30"(w109) -> ()
              n506 = local write "A_31"(w109) -> ()
              n507 = local write "A_32"(w109) -> ()
              n508 = local write "A_25"(w109) -> ()
              n509 = local write "A_26"(w109) -> ()
              n510 = local write "A_24"(w109) -> ()
              n511 = local write "A_17"(w109) -> ()
              n512 = local write "A_18"(w109) -> ()
              n513 = local write "A_19"(w109) -> ()
              n514 = local write "A_20"(w109) -> ()
              n515 = local write "A_21"(w109) -> ()
              n516 = local write "A_22"(w109) -> ()
              n517 = local write "A_23"(w109) -> ()
            }
            frame 14 {
              w110 = TRUE
              w111 = FALSE
              n518 = local write "A_10"(w110) -> ()
              n519 = local write "A_11"(w110) -> ()
              n520 = local write "A_12"(w110) -> ()
              n521 = local write "A_13"(w110) -> ()
              n522 = local write "A_14"(w110) -> ()
              n523 = local write "A_15"(w111) -> ()
              n524 = local write "A_16"(w111) -> ()
              n525 = local write "A_1"(w110) -> ()
              n526 = local write "A_2"(w110) -> ()
              n527 = local write "A_3"(w110) -> ()
              n528 = local write "A_4"(w110) -> ()
              n529 = local write "A_5"(w110) -> ()
              n530 = local write "A_6"(w110) -> ()
              n531 = local write "A_7"(w110) -> ()
              n532 = local write "A_8"(w110) -> ()
              n533 = local write "A_9"(w110) -> ()
              n534 = local write "A_27"(w111) -> ()
              n535 = local write "A_28"(w111) -> ()
              n536 = local write "A_29"(w111) -> ()
              n537 = local write "A_30"(w111) -> ()
              n538 = local write "A_31"(w111) -> ()
              n539 = local write "A_32"(w111) -> ()
              n540 = local write "A_25"(w111) -> ()
              n541 = local write "A_26"(w111) -> ()
              n542 = local write "A_24"(w111) -> ()
              n543 = local write "A_17"(w111) -> ()
              n544 = local write "A_18"(w111) -> ()
              n545 = local write "A_19"(w111) -> ()
              n546 = local write "A_20"(w111) -> ()
              n547 = local write "A_21"(w111) -> ()
              n548 = local write "A_22"(w111) -> ()
              n549 = local write "A_23"(w111) -> ()
            }
            frame 15 {
              w112 = TRUE
              w113 = FALSE
              n550 = local write "A_10"(w112) -> ()
              n551 = local write "A_11"(w112) -> ()
              n552 = local write "A_12"(w112) -> ()
              n553 = local write "A_13"(w112) -> ()
              n554 = local write "A_14"(w112) -> ()
              n555 = local write "A_15"(w112) -> ()
              n556 = local write "A_16"(w113) -> ()
              n557 = local write "A_1"(w112) -> ()
              n558 = local write "A_2"(w112) -> ()
              n559 = local write "A_3"(w112) -> ()
              n560 = local write "A_4"(w112) -> ()
              n561 = local write "A_5"(w112) -> ()
              n562 = local write "A_6"(w112) -> ()
              n563 = local write "A_7"(w112) -> ()
              n564 = local write "A_8"(w112) -> ()
              n565 = local write "A_9"(w112) -> ()
              n566 = local write "A_27"(w113) -> ()
              n567 = local write "A_28"(w113) -> ()
              n568 = local write "A_29"(w113) -> ()
              n569 = local write "A_30"(w113) -> ()
              n570 = local write "A_31"(w113) -> ()
              n571 = local write "A_32"(w113) -> ()
              n572 = local write "A_25"(w113) -> ()
              n573 = local write "A_26"(w113) -> ()
              n574 = local write "A_24"(w113) -> ()
              n575 = local write "A_17"(w113) -> ()
              n576 = local write "A_18"(w113) -> ()
              n577 = local write "A_19"(w113) -> ()
              n578 = local write "A_20"(w113) -> ()
              n579 = local write "A_21"(w113) -> ()
              n580 = local write "A_22"(w113) -> ()
              n581 = local write "A_23"(w113) -> ()
            }
            frame 16 {
              w114 = TRUE
              w115 = FALSE
              n582 = local write "A_10"(w114) -> ()
              n583 = local write "A_11"(w114) -> ()
              n584 = local write "A_12"(w114) -> ()
              n585 = local write "A_13"(w114) -> ()
              n586 = local write "A_14"(w114) -> ()
              n587 = local write "A_15"(w114) -> ()
              n588 = local write "A_16"(w114) -> ()
              n589 = local write "A_1"(w114) -> ()
              n590 = local write "A_2"(w114) -> ()
              n591 = local write "A_3"(w114) -> ()
              n592 = local write "A_4"(w114) -> ()
              n593 = local write "A_5"(w114) -> ()
              n594 = local write "A_6"(w114) -> ()
              n595 = local write "A_7"(w114) -> ()
              n596 = local write "A_8"(w114) -> ()
              n597 = local write "A_9"(w114) -> ()
              n598 = local write "A_27"(w115) -> ()
              n599 = local write "A_28"(w115) -> ()
              n600 = local write "A_29"(w115) -> ()
              n601 = local write "A_30"(w115) -> ()
              n602 = local write "A_31"(w115) -> ()
              n603 = local write "A_32"(w115) -> ()
              n604 = local write "A_25"(w115) -> ()
              n605 = local write "A_26"(w115) -> ()
              n606 = local write "A_24"(w115) -> ()
              n607 = local write "A_17"(w115) -> ()
              n608 = local write "A_18"(w115) -> ()
              n609 = local write "A_19"(w115) -> ()
              n610 = local write "A_20"(w115) -> ()
              n611 = local write "A_21"(w115) -> ()
              n612 = local write "A_22"(w115) -> ()
              n613 = local write "A_23"(w115) -> ()
            }
          }
        }
      }
    }
    frame #1 {
      w118 = "Type2_ANumCheck" ("名称（未命名）")
      w120 = "Type2_ANumCheck" ("名称（未命名）")
      n614 = while {
        stop <- w372 stop-if-true
        n615 = event shown="[3] \"btn_全选\": 值改变" {
          selector: _ -> [_ _ _ _ _ _]
          dyn-events: _ -> [_ _ _ _ _ _]
          timeout: _ -> [_ _ _ _ _ _]
          tunnel: [_ TRUE _ _ _ TRUE] -> w372
          event Timeout {
            n616 = event-data() -> ()  [unwired: 1 in, 2 out]
          }
          event Panel Close {
            n617 = event-data() -> ()  [unwired: 1 in, 3 out]
          }
          event "btn_开始测试": Value Change {
            n618 = event-data() -> ()  [unwired: 1 in, 5 out]
            n619 = stacked-sequence {
              frame #0 {
                # "测试期间不准退出防止程序卡死"
                n620 = local read "Analog_back"() -> (w374:string[][])
                n621 = for {
                  tunnel: w374 -> [w378] mode=indexing
                  i -> [w377]
                  n622 = for {
                    tunnel: w378 -> [_] mode=indexing
                    tunnel: w377 -> [w380]
                    i -> [w379]
                    n623 = local read "Analog_back"() -> (w383:string[][])
                    n624 = Replace Array Subset(array=w383, new element="", index (row)=w380, index (col)=w379) -> (w382:string[][])
                    n625 = local write "Analog_back"(w382) -> ()
                  }
                }
                n626 = for {
                  N: 32 -> [_]
                  i -> [w385]
                  n627 = case shown="2" w385 {
                    tunnel: cluster{u32, u32}[] [{9868950, 9868950}] -> [w386 w387 w388 w389 w390 w391 w392 w393 w394 w395 w396 w397 w398 w399 w400 w401 w402 w403 w404 w405 w406 w407 w408 w409 w410 w411 w412 w413 w414 w415 w416 w417]
                    frame 0, Default {
                      n628 = property on="light_1" class="Bool (严格)"("Colors [4]"=w386) -> ()  [unwired: 2 in, 2 out]
                    }
                    frame 1 {
                      n629 = property on="light_2" class="Bool (严格)"("Colors [4]"=w387) -> ()  [unwired: 2 in, 2 out]
                    }
                    frame 2 {
                      n630 = property on="light_3" class="Bool (严格)"("Colors [4]"=w388) -> ()  [unwired: 2 in, 2 out]
                    }
                    frame 3 {
                      n631 = property on="light_4" class="Bool (严格)"("Colors [4]"=w389) -> ()  [unwired: 2 in, 2 out]
                    }
                    frame 4 {
                      n632 = property on="light_5" class="Bool (严格)"("Colors [4]"=w390) -> ()  [unwired: 2 in, 2 out]
                    }
                    frame 5 {
                      n633 = property on="light_6" class="Bool (严格)"("Colors [4]"=w391) -> ()  [unwired: 2 in, 2 out]
                    }
                    frame 6 {
                      n634 = property on="light_7" class="Bool (严格)"("Colors [4]"=w392) -> ()  [unwired: 2 in, 2 out]
                    }
                    frame 7 {
                      n635 = property on="light_8" class="Bool (严格)"("Colors [4]"=w393) -> ()  [unwired: 2 in, 2 out]
                    }
                    frame 8 {
                      n636 = property on="light_9" class="Bool (严格)"("Colors [4]"=w394) -> ()  [unwired: 2 in, 2 out]
                    }
                    frame 9 {
                      n637 = property on="light_10" class="Bool (严格)"("Colors [4]"=w395) -> ()  [unwired: 2 in, 2 out]
                    }
                    frame 10 {
                      n638 = property on="light_11" class="Bool (严格)"("Colors [4]"=w396) -> ()  [unwired: 2 in, 2 out]
                    }
                    frame 11 {
                      n639 = property on="light_12" class="Bool (严格)"("Colors [4]"=w397) -> ()  [unwired: 2 in, 2 out]
                    }
                    frame 12 {
                      n640 = property on="light_13" class="Bool (严格)"("Colors [4]"=w398) -> ()  [unwired: 2 in, 2 out]
                    }
                    frame 13 {
                      n641 = property on="light_14" class="Bool (严格)"("Colors [4]"=w399) -> ()  [unwired: 2 in, 2 out]
                    }
                    frame 14 {
                      n642 = property on="light_15" class="Bool (严格)"("Colors [4]"=w400) -> ()  [unwired: 2 in, 2 out]
                    }
                    frame 15 {
                      n643 = property on="light_16" class="Bool (严格)"("Colors [4]"=w401) -> ()  [unwired: 2 in, 2 out]
                    }
                    frame 16 {
                      n644 = property on="light_17" class="Bool (严格)"("Colors [4]"=w402) -> ()  [unwired: 2 in, 2 out]
                    }
                    frame 17 {
                      n645 = property on="light_18" class="Bool (严格)"("Colors [4]"=w403) -> ()  [unwired: 2 in, 2 out]
                    }
                    frame 18 {
                      n646 = property on="light_19" class="Bool (严格)"("Colors [4]"=w404) -> ()  [unwired: 2 in, 2 out]
                    }
                    frame 19 {
                      n647 = property on="light_20" class="Bool (严格)"("Colors [4]"=w405) -> ()  [unwired: 2 in, 2 out]
                    }
                    frame 20 {
                      n648 = property on="light_21" class="Bool (严格)"("Colors [4]"=w406) -> ()  [unwired: 2 in, 2 out]
                    }
                    frame 21 {
                      n649 = property on="light_22" class="Bool (严格)"("Colors [4]"=w407) -> ()  [unwired: 2 in, 2 out]
                    }
                    frame 22 {
                      n650 = property on="light_23" class="Bool (严格)"("Colors [4]"=w408) -> ()  [unwired: 2 in, 2 out]
                    }
                    frame 23 {
                      n651 = property on="light_24" class="Bool (严格)"("Colors [4]"=w409) -> ()  [unwired: 2 in, 2 out]
                    }
                    frame 24 {
                      n652 = property on="light_25" class="Bool (严格)"("Colors [4]"=w410) -> ()  [unwired: 2 in, 2 out]
                    }
                    frame 25 {
                      n653 = property on="light_26" class="Bool (严格)"("Colors [4]"=w411) -> ()  [unwired: 2 in, 2 out]
                    }
                    frame 26 {
                      n654 = property on="light_27" class="Bool (严格)"("Colors [4]"=w412) -> ()  [unwired: 2 in, 2 out]
                    }
                    frame 27 {
                      n655 = property on="light_28" class="Bool (严格)"("Colors [4]"=w413) -> ()  [unwired: 2 in, 2 out]
                    }
                    frame 28 {
                      n656 = property on="light_29" class="Bool (严格)"("Colors [4]"=w414) -> ()  [unwired: 2 in, 2 out]
                    }
                    frame 29 {
                      n657 = property on="light_30" class="Bool (严格)"("Colors [4]"=w415) -> ()  [unwired: 2 in, 2 out]
                    }
                    frame 30 {
                      n658 = property on="light_31" class="Bool (严格)"("Colors [4]"=w416) -> ()  [unwired: 2 in, 2 out]
                    }
                    frame 31 {
                      n659 = property on="light_32" class="Bool (严格)"("Colors [4]"=w417) -> ()  [unwired: 2 in, 2 out]
                    }
                  }
                }
                n660 = property on="btn_取消" class="Bool"("DisabledEnum"=T1."Disabled and Grayed Out" ("禁用")) -> ()  [unwired: 2 in, 2 out]
              }
              frame #1 {
                n661 = for {
                  N: 32 -> [_]
                  i -> [w420]
                  n662 = for {
                    N: 7 -> [_]
                    tunnel: w420 -> [w427]
                    i -> [w424]
                    n663 = Quotient & Remainder(x=w427, y=2) -> (x-y*floor(x/y)=w425:i32)  [unwired: 1 out]
                    n664 = Equal To 0?(x=w425) -> (x = 0?=w428:bool)
                    n665 = case shown="真" w428 {
                      tunnel: [u32 16448250 u32 15723488] -> w421
                      frame False {
                      }
                      frame True {
                      }
                    }
                    n666 = Bundle(w427, w424) -> (w423:cluster{i32, i32})  [unwired: 1 in]
                    n667 = property on="Analog_back" class="Tbl (严格)"("Active Cell"=w423) -> (error out=w422:errorcluster)  [unwired: 2 in, 1 out]
                    n668 = property on="Analog_back" class="Tbl (严格)"(error in=w422, "Cell BG Color"=w421) -> ()  [unwired: 1 in, 2 out]
                  }
                }
              }
              frame #2 {
                w443 = -99
                w442 = FALSE
                n669 = Initialize Array(TRUE, 32 ("维数大小"), 2 ("维数大小")) -> (w438:bool[][])
                n670 = local write "记录跳变次数"(0) -> ()
                n671 = local write "发送值状态"(1 ("发送值状态")) -> ()
                n672 = local write "反馈值"(1) -> ()
                n673 = local write "最近一次跳变防线值"(w443) -> ()
                n674 = local write "当前波动值"(w443) -> ()
                n675 = local write "合格？"(w438) -> ()
                n676 = local write "第几组数据"(0 ("第几组数据")) -> ()
                n677 = local write "bSend"(w442) -> ()
                n678 = local write "bRecv"(w442) -> ()
                n679 = Initialize Array("", 32 ("维数大小"), 3 ("维数大小")) -> (w434:string[][])
                n680 = local write "Analog_IN"(w434) -> ()
              }
              frame #3 {
                n681 = local read "A_10"() -> (w468:bool)
                n682 = local read "A_11"() -> (w467:bool)
                n683 = local read "A_12"() -> (w466:bool)
                n684 = local read "A_13"() -> (w465:bool)
                n685 = local read "A_14"() -> (w464:bool)
                n686 = local read "A_15"() -> (w463:bool)
                n687 = local read "A_16"() -> (w462:bool)
                n688 = local read "A_17"() -> (w461:bool)
                n689 = local read "A_18"() -> (w460:bool)
                n690 = local read "A_19"() -> (w459:bool)
                n691 = local read "A_20"() -> (w458:bool)
                n692 = local read "A_21"() -> (w457:bool)
                n693 = local read "A_22"() -> (w456:bool)
                n694 = local read "A_23"() -> (w455:bool)
                n695 = local read "A_24"() -> (w454:bool)
                n696 = local read "A_25"() -> (w453:bool)
                n697 = local read "A_26"() -> (w452:bool)
                n698 = local read "A_27"() -> (w451:bool)
                n699 = local read "A_28"() -> (w450:bool)
                n700 = local read "A_29"() -> (w449:bool)
                n701 = local read "A_30"() -> (w448:bool)
                n702 = local read "A_31"() -> (w447:bool)
                n703 = local read "A_32"() -> (w446:bool)
                n704 = local read "A_1"() -> (w477:bool)
                n705 = local read "A_2"() -> (w476:bool)
                n706 = local read "A_3"() -> (w475:bool)
                n707 = local read "A_4"() -> (w474:bool)
                n708 = local read "A_5"() -> (w473:bool)
                n709 = local read "A_6"() -> (w472:bool)
                n710 = local read "A_7"() -> (w471:bool)
                n711 = local read "A_8"() -> (w470:bool)
                n712 = local read "A_9"() -> (w469:bool)
                n713 = Build Array(w477, w476, w475, w474, w473, w472, w471, w470, w469, w468, w467, w466, w465, w464, w463, w462, w461, w460, w459, w458, w457, w456, w455, w454, w453, w452, w451, w450, w449, w448, w447, w446) -> (w478:bool[])
                n714 = Or Array Elements(Boolean array=w478) -> (logical OR=w445:bool)
                n715 = local write "数组_选择"(w478) -> ()
                n716 = case shown="真" w445 {
                  frame False {
                    n717 = call "显示对话框信息"() -> ()  [unwired: 10 in, 2 out]
                  }
                  frame True {
                    n718 = local write "starttest"(TRUE) -> ()
                  }
                }
              }
            }
          }
          event "btn_全选": Value Change {
            w480 = TRUE
            n719 = event-data() -> ()  [unwired: 1 in, 5 out]
            n720 = local write "A_10"(w480) -> ()
            n721 = local write "A_11"(w480) -> ()
            n722 = local write "A_12"(w480) -> ()
            n723 = local write "A_13"(w480) -> ()
            n724 = local write "A_14"(w480) -> ()
            n725 = local write "A_15"(w480) -> ()
            n726 = local write "A_16"(w480) -> ()
            n727 = local write "A_1"(w480) -> ()
            n728 = local write "A_2"(w480) -> ()
            n729 = local write "A_3"(w480) -> ()
            n730 = local write "A_4"(w480) -> ()
            n731 = local write "A_5"(w480) -> ()
            n732 = local write "A_6"(w480) -> ()
            n733 = local write "A_7"(w480) -> ()
            n734 = local write "A_8"(w480) -> ()
            n735 = local write "A_9"(w480) -> ()
            n736 = local write "A_27"(w480) -> ()
            n737 = local write "A_28"(w480) -> ()
            n738 = local write "A_29"(w480) -> ()
            n739 = local write "A_30"(w480) -> ()
            n740 = local write "A_31"(w480) -> ()
            n741 = local write "A_32"(w480) -> ()
            n742 = local write "A_25"(w480) -> ()
            n743 = local write "A_26"(w480) -> ()
            n744 = local write "A_24"(w480) -> ()
            n745 = local write "A_17"(w480) -> ()
            n746 = local write "A_18"(w480) -> ()
            n747 = local write "A_19"(w480) -> ()
            n748 = local write "A_20"(w480) -> ()
            n749 = local write "A_21"(w480) -> ()
            n750 = local write "A_22"(w480) -> ()
            n751 = local write "A_23"(w480) -> ()
          }
          event "btn_反选": Value Change {
            n752 = event-data() -> ()  [unwired: 1 in, 5 out]
            n753 = local read "A_10"() -> (w531:bool)
            n754 = local read "A_11"() -> (w530:bool)
            n755 = local read "A_12"() -> (w529:bool)
            n756 = local read "A_13"() -> (w528:bool)
            n757 = local read "A_14"() -> (w527:bool)
            n758 = local read "A_15"() -> (w526:bool)
            n759 = local read "A_16"() -> (w525:bool)
            n760 = local read "A_1"() -> (w544:bool)
            n761 = local read "A_2"() -> (w542:bool)
            n762 = local read "A_3"() -> (w540:bool)
            n763 = local read "A_4"() -> (w537:bool)
            n764 = local read "A_5"() -> (w536:bool)
            n765 = local read "A_6"() -> (w535:bool)
            n766 = local read "A_7"() -> (w534:bool)
            n767 = local read "A_8"() -> (w533:bool)
            n768 = local read "A_9"() -> (w532:bool)
            n769 = Not(x=w544) -> (.not. x?=w543:bool)
            n770 = Not(x=w542) -> (.not. x?=w541:bool)
            n771 = Not(x=w540) -> (.not. x?=w539:bool)
            n772 = Not(x=w537) -> (.not. x?=w538:bool)
            n773 = Not(x=w536) -> (.not. x?=w524:bool)
            n774 = Not(x=w535) -> (.not. x?=w523:bool)
            n775 = Not(x=w534) -> (.not. x?=w522:bool)
            n776 = Not(x=w533) -> (.not. x?=w521:bool)
            n777 = Not(x=w532) -> (.not. x?=w520:bool)
            n778 = Not(x=w531) -> (.not. x?=w519:bool)
            n779 = Not(x=w530) -> (.not. x?=w518:bool)
            n780 = Not(x=w529) -> (.not. x?=w517:bool)
            n781 = Not(x=w528) -> (.not. x?=w516:bool)
            n782 = Not(x=w527) -> (.not. x?=w515:bool)
            n783 = Not(x=w526) -> (.not. x?=w514:bool)
            n784 = Not(x=w525) -> (.not. x?=w513:bool)
            n785 = local write "A_1"(w543) -> ()
            n786 = local write "A_2"(w541) -> ()
            n787 = local write "A_3"(w539) -> ()
            n788 = local write "A_4"(w538) -> ()
            n789 = local write "A_5"(w524) -> ()
            n790 = local write "A_6"(w523) -> ()
            n791 = local write "A_7"(w522) -> ()
            n792 = local write "A_8"(w521) -> ()
            n793 = local write "A_9"(w520) -> ()
            n794 = local write "A_10"(w519) -> ()
            n795 = local write "A_11"(w518) -> ()
            n796 = local write "A_12"(w517) -> ()
            n797 = local write "A_13"(w516) -> ()
            n798 = local write "A_14"(w515) -> ()
            n799 = local write "A_15"(w514) -> ()
            n800 = local write "A_16"(w513) -> ()
            n801 = local read "A_27"() -> (w491:bool)
            n802 = local read "A_28"() -> (w489:bool)
            n803 = local read "A_29"() -> (w487:bool)
            n804 = local read "A_30"() -> (w485:bool)
            n805 = local read "A_31"() -> (w483:bool)
            n806 = local read "A_32"() -> (w481:bool)
            n807 = local read "A_25"() -> (w495:bool)
            n808 = local read "A_26"() -> (w493:bool)
            n809 = local read "A_24"() -> (w497:bool)
            n810 = local read "A_17"() -> (w511:bool)
            n811 = local read "A_18"() -> (w509:bool)
            n812 = local read "A_19"() -> (w507:bool)
            n813 = local read "A_20"() -> (w505:bool)
            n814 = local read "A_21"() -> (w502:bool)
            n815 = local read "A_22"() -> (w501:bool)
            n816 = local read "A_23"() -> (w498:bool)
            n817 = Not(x=w491) -> (.not. x?=w490:bool)
            n818 = Not(x=w489) -> (.not. x?=w488:bool)
            n819 = Not(x=w487) -> (.not. x?=w486:bool)
            n820 = Not(x=w485) -> (.not. x?=w484:bool)
            n821 = Not(x=w483) -> (.not. x?=w482:bool)
            n822 = Not(x=w481) -> (.not. x?=w512:bool)
            n823 = Not(x=w495) -> (.not. x?=w494:bool)
            n824 = Not(x=w493) -> (.not. x?=w492:bool)
            n825 = Not(x=w497) -> (.not. x?=w496:bool)
            n826 = Not(x=w511) -> (.not. x?=w510:bool)
            n827 = Not(x=w509) -> (.not. x?=w508:bool)
            n828 = Not(x=w507) -> (.not. x?=w506:bool)
            n829 = Not(x=w505) -> (.not. x?=w504:bool)
            n830 = Not(x=w502) -> (.not. x?=w503:bool)
            n831 = Not(x=w501) -> (.not. x?=w500:bool)
            n832 = Not(x=w498) -> (.not. x?=w499:bool)
            n833 = local write "A_27"(w490) -> ()
            n834 = local write "A_28"(w488) -> ()
            n835 = local write "A_29"(w486) -> ()
            n836 = local write "A_30"(w484) -> ()
            n837 = local write "A_31"(w482) -> ()
            n838 = local write "A_32"(w512) -> ()
            n839 = local write "A_25"(w494) -> ()
            n840 = local write "A_26"(w492) -> ()
            n841 = local write "A_24"(w496) -> ()
            n842 = local write "A_17"(w510) -> ()
            n843 = local write "A_18"(w508) -> ()
            n844 = local write "A_19"(w506) -> ()
            n845 = local write "A_20"(w504) -> ()
            n846 = local write "A_21"(w503) -> ()
            n847 = local write "A_22"(w500) -> ()
            n848 = local write "A_23"(w499) -> ()
          }
          event "btn_取消": Value Change {
            n849 = event-data() -> ()  [unwired: 1 in, 5 out]
          }
        }
        n850 = local write "退出？"(w372) -> ()
      }
      n851 = Obtain Notifier(name (unnamed)=w120, notification data type=w120) -> (notifier out=w119:refnum<notifier>)  [unwired: 2 in, 2 out]
      n852 = while {
        tunnel: w119 -> [w274]
        stop <- w277 stop-if-true
        n853 = local read "starttest"() -> (w276:bool)
        n854 = Wait Until Next ms Multiple(millisecond multiple=u32 10 ("毫秒倍数")) -> ()  [unwired: 1 out]
        n855 = case shown="真" w276 {
          tunnel: w274 -> [_ w278]
          frame False {
          }
          frame True {
            n856 = stacked-sequence {
              tunnel: w278 -> [w279 _]
              frame #0 {
                n857 = for {
                  N: 32 -> [_]
                  tunnel: w279 -> [w281]
                  i -> [w282]
                  n858 = local read "数组_选择"() -> (w284:bool[])
                  n859 = local write "第几组数据"(w282) -> ()
                  n860 = Index Array(array=w284, index=w282) -> (element=w283:bool)
                  n861 = case shown="真" w283 {
                    tunnel: w282 -> [_ w286]
                    tunnel: w281 -> [_ w285]
                    frame False {
                    }
                    frame True {
                      n862 = global read "试验配置信息.vi" "输出切换ID"() -> (w289:i32[])
                      n863 = global read "试验配置信息.vi" "输入切换ID"() -> (w290:i32[])
                      n864 = Index Array(array=w289, index=w286) -> (element=w288:i32)
                      n865 = Index Array(array=w290, index=w286) -> (element=w291:i32)
                      n866 = call "can开关切换.vi"("输入切换ID"=w291, "输出切换ID"=w288, "函数类型"=2) -> ()  [unwired: 7 in, 1 out]
                      n867 = case shown="真" TRUE {
                        tunnel: w286 -> [w293 _]
                        tunnel: w285 -> [_ w297]
                        frame False {
                          n868 = Increment(x=w293) -> (x+1=w296:i32)
                          n869 = Format Into String(format string="第%d路CAN切换失败！", w296) -> (resulting string=w295:string)  [unwired: 2 in, 1 out]
                          n870 = call "显示对话框信息2"("Message"=w295) -> ()  [unwired: 9 in, 2 out]
                        }
                        frame True {
                          n871 = stacked-sequence {
                            tunnel: w297 -> [_ w302]
                            frame #0 {
                              w299 = -99
                              # "每次在发新一组数据时，都初始化"
                              n872 = local write "记录跳变次数"(0) -> ()
                              n873 = local write "发送值状态"(1 ("发送值状态")) -> ()
                              n874 = local write "反馈值"(1) -> ()
                              n875 = local write "最近一次跳变防线值"(w299) -> ()
                              n876 = local write "当前波动值"(w299) -> ()
                            }
                            frame #1 {
                              n877 = while {
                                tunnel: w302 -> [w304]
                                stop <- w303 stop-if-true
                                n878 = local read "bSend"() -> (w306:bool)
                                n879 = Not(x=w306) -> (.not. x?=w305:bool)
                                n880 = case shown="真" w305 {
                                tunnel: w304 -> [_ w319]
                                tunnel: [w307 FALSE] -> w303
                                frame False {
                                # "数据已发送 判断回包是否已收到"
                                n881 = local read "bRecv"() -> (w308:bool)
                                n882 = case shown="真" w308 {
                                tunnel: [FALSE w310] -> w307
                                frame False {
                                }
                                frame True {
                                n883 = local read "发送值状态"() -> (w313:i32)
                                n884 = Equal?(x=w313, y=3) -> (x = y?=w311:bool)
                                n885 = case shown="假" w311 {
                                tunnel: [w314 TRUE] -> w310
                                frame False {
                                n886 = stacked-sequence {
                                tunnel: [_ FALSE] -> w314
                                frame #0 {
                                w315 = FALSE
                                n887 = local write "bSend"(w315) -> ()
                                n888 = local write "bRecv"(w315) -> ()
                                }
                                frame #1 {
                                }
                                }
                                }
                                frame True {
                                # "判断当前数据是否已发送完毕"
                                }
                                }
                                }
                                }
                                }
                                frame True {
                                n889 = stacked-sequence {
                                tunnel: w319 -> [_ _ _ w367 _]
                                frame #0 {
                                n890 = Wait Until Next ms Multiple(millisecond multiple=u32 100 ("毫秒倍数")) -> ()  [unwired: 1 out]
                                }
                                frame #1 {
                                n891 = local read "发送值"() -> (w323:dbl)
                                n892 = Equal?(x=w323, y=-99.0) -> (x = y?=w321:bool)
                                n893 = case shown="假" w321 {
                                frame False {
                                n894 = local read "发送值状态"() -> (w324:i32)
                                n895 = case shown="2" w324 {
                                frame 1, Default {
                                # "当前状态是递增"
                                n896 = stacked-sequence {
                                frame #0 {
                                n897 = local read "发送值"() -> (w327:dbl)
                                n898 = local read "变化量"() -> (w326:dbl)
                                n899 = Add(x=w327, y=w326) -> (x+y=w325:dbl)
                                n900 = local write "发送值"(w325) -> ()
                                }
                                frame #1 {
                                n901 = local read "第几组数据"() -> (w330:i32)
                                n902 = global read "试验配置信息.vi" "Max"() -> (w331:dbl[])
                                n903 = local read "发送值"() -> (w332:dbl)
                                n904 = Index Array(array=w331, index=w330) -> (element=w328:dbl)
                                n905 = Greater Or Equal?(x=w332, y=w328) -> (x >= y?=w329:bool)
                                n906 = case shown="真" w329 {
                                tunnel: w328 -> [_ w334]
                                frame False {
                                }
                                frame True {
                                # "超过最大值时\n将状态改为递减状态"
                                n907 = local write "发送值"(w334) -> ()
                                n908 = local write "发送值状态"(2 ("y")) -> ()
                                }
                                }
                                }
                                }
                                }
                                frame 2 {
                                # "当前状态为递减状态"
                                n909 = stacked-sequence {
                                frame #0 {
                                n910 = local read "发送值"() -> (w337:dbl)
                                n911 = local read "变化量"() -> (w336:dbl)
                                n912 = Subtract(x=w337, y=w336) -> (x-y=w335:dbl)
                                n913 = local write "发送值"(w335) -> ()
                                }
                                frame #1 {
                                n914 = local read "第几组数据"() -> (w340:i32)
                                n915 = global read "试验配置信息.vi" "min"() -> (w341:dbl[])
                                n916 = local read "发送值"() -> (w342:dbl)
                                n917 = Index Array(array=w341, index=w340) -> (element=w338:dbl)
                                n918 = Less Or Equal?(x=w342, y=w338) -> (x <= y?=w339:bool)
                                n919 = case shown="真" w339 {
                                tunnel: w338 -> [_ w344]
                                frame False {
                                }
                                frame True {
                                # "递减到最小值时 代表发送了一个周期"
                                n920 = local write "发送值"(w344) -> ()
                                n921 = local write "发送值状态"(3) -> ()
                                }
                                }
                                }
                                }
                                }
                                }
                                }
                                frame True {
                                # "默认值 证明为发送的第一条数据\n从最小值开始"
                                n922 = local read "第几组数据"() -> (w346:i32)
                                n923 = global read "试验配置信息.vi" "min"() -> (w347:dbl[])
                                n924 = Index Array(array=w347, index=w346) -> (element=w345:dbl)
                                n925 = local write "发送值"(w345) -> ()
                                }
                                }
                                }
                                frame #2 {
                                # "KwgfrW031h"
                                # "PCI板卡下发模拟量数据"
                                n926 = local read "第几组数据"() -> (w359:i32)
                                n927 = global read "试验配置信息.vi" "设定输出通道"() -> (w360:i32[])
                                n928 = local read "发送值"() -> (w348:dbl)
                                n929 = To Long Integer(number=w359) -> (32bit integer=w350:i32)
                                n930 = local read "发送值"() -> (w358:dbl)
                                n931 = Index Array(array=w360, index=w350) -> (element=w349:i32)
                                n932 = Number To Fractional String(number=w348, precision (6)=i16 3 ("精度(6)")) -> (F-format string=w352:string)  [unwired: 2 in]
                                n933 = case shown="1" w349 {
                                tunnel: [w363 w366] -> w356
                                tunnel: w358 -> [w361 w364]
                                frame 0, Default {
                                n934 = Build Array(w361, 0.0) -> (w363:dbl[])
                                }
                                frame 1 {
                                n935 = Build Array(0.0, w364) -> (w366:dbl[])
                                }
                                }
                                n936 = local read "Analog_IN"() -> (w355:string[][])
                                n937 = Replace Array Subset(array=w355, new element=w352, index (row)=w350, index (col)=2 ("禁用的索引 (列)")) -> (w354:string[][])
                                n938 = call "Convert to Dynamic Data"("Array"=w356) -> ("Dynamic Data Type"=w357:dynamicdata)  [unwired: 3 out]
                                n939 = local write "Analog_IN"(w354) -> ()
                                n940 = call "DAQNavi Assistant"("data in(DDT)"=w357) -> ()  [unwired: 2 in, 17 out]
                                }
                                frame #3 {
                                n941 = Send Notification(notification="NumCheck" ("通知"), notifier=w367) -> ()  [unwired: 1 in, 2 out]
                                }
                                frame #4 {
                                n942 = local write "bSend"(TRUE) -> ()
                                }
                                }
                                }
                                }
                              }
                            }
                          }
                        }
                      }
                    }
                  }
                }
              }
              frame #1 {
                n943 = local write "starttest"(FALSE) -> ()
                n944 = property on="btn_取消" class="Bool"("DisabledEnum"=T1."Enabled" ("禁用")) -> ()  [unwired: 2 in, 2 out]
              }
            }
          }
        }
        n945 = local read "退出？"() -> (w277:bool)
      }
      n946 = Obtain Notifier(name (unnamed)=w118, notification data type=w118) -> (notifier out=w117:refnum<notifier>)  [unwired: 2 in, 2 out]
      n947 = while {
        tunnel: w117 -> [w126]
        tunnel: [w125] -> w116
        stop <- w128 stop-if-true
        n948 = Wait Until Next ms Multiple(millisecond multiple=u32 10 ("毫秒倍数")) -> ()  [unwired: 1 out]
        n949 = Wait on Notification(notifier=w126, timeout in ms (-1)=10 ("超时毫秒(-1)")) -> (notifier out=w125:refnum<notifier>, notification=w124:string)  [unwired: 2 in, 2 out]
        n950 = Equal?(x=w124, y="NumCheck" ("通知")) -> (x = y?=w122:bool)
        n951 = case shown="真" w122 {
          frame False {
          }
          frame True {
            n952 = stacked-sequence {
              frame #0 {
                n953 = local read "第几组数据"() -> (w130:i32)
                n954 = global read "试验配置信息.vi" "设定输入通道"() -> (w132:i32[])
                n955 = Index Array(array=w132, index=w130) -> (element=w131:i32)
                n956 = call "DAQNavi Assistant2"() -> ("dataOut(U8Array)"=w133:u8[])  [unwired: 2 in, 17 out]
                n957 = Index Array(array=w133, index #1=0 ("索引"), index #2=1 ("索引")) -> (element #1=w138:u8, element #2=w139:u8)
                n958 = Number To Boolean Array(number=w138) -> (Boolean array=w134:bool[])
                n959 = Number To Boolean Array(number=w139) -> (Boolean array=w135:bool[])
                n960 = Build Array (concatenate)(w134, w135) -> (w140:bool[])
                n961 = Boolean To (0,1) ("布尔值至(0,1)转换")(Boolean=w140) -> (0, 1=w141:i16[])
                n962 = Index Array(array=w141, index=w131) -> (element=w129:i16)
                n963 = local write "反馈值"(w129) -> ()
              }
              frame #1 {
                n964 = local read "最近一次跳变防线值"() -> (w144:i32)
                n965 = Equal?(x=w144, y=-99) -> (x = y?=w143:bool)
                n966 = case shown="假" w143 {
                  frame False {
                    # "当前值与上次值不同，则发生跳变"
                    n967 = local read "最近一次跳变防线值"() -> (w146:i32)
                    n968 = local read "反馈值"() -> (w147:i32)
                    n969 = Equal?(x=w147, y=w146) -> (x = y?=w145:bool)
                    n970 = case shown="真" w145 {
                      frame False {
                      }
                      frame True {
                        n971 = stacked-sequence {
                          frame #0 {
                            n972 = local read "反馈值"() -> (w150:i32)
                            n973 = local read "记录跳变次数"() -> (w149:i32)
                            n974 = Increment(x=w149) -> (x+1=w148:i32)
                            n975 = local write "最近一次跳变防线值"(w150) -> ()
                            n976 = local write "记录跳变次数"(w148) -> ()
                          }
                          frame #1 {
                            n977 = local read "记录跳变次数"() -> (w151:i32)
                            n978 = case shown="1, 默认" w151 {
                              frame 1, Default {
                                n979 = local read "第几组数据"() -> (w159:i32)
                                n980 = global read "试验配置信息.vi" "允许误差"() -> (w176:dbl[])
                                n981 = global read "试验配置信息.vi" "参数A1"() -> (w175:dbl[])
                                n982 = global read "试验配置信息.vi" "Max"() -> (w172:dbl[])
                                n983 = global read "试验配置信息.vi" "min"() -> (w171:dbl[])
                                n984 = local read "发送值"() -> (w155:dbl)
                                n985 = local read "最近一次跳变防线值"() -> (w154:i32)
                                n986 = Index Array(array=w175, index=w159) -> (element=w174:dbl)
                                n987 = Index Array(array=w172, index=w159) -> (element=w169:dbl)
                                n988 = Index Array(array=w171, index=w159) -> (element=w168:dbl)
                                n989 = Index Array(array=w176, index=w159) -> (element=w173:dbl)
                                n990 = Subtract(x=w169, y=w168) -> (x-y=w170:dbl)
                                n991 = Absolute Value(x=w170) -> (abs(x)=w167:dbl)
                                n992 = local read "数组_选择"() -> (w166:bool[])
                                n993 = local read "第几组数据"() -> (w156:i32)
                                n994 = Equal To 0?(x=w154) -> (x = 0?=w178:bool)
                                n995 = Number To Fractional String(number=w155, precision (6)=i16 3 ("精度(6)")) -> (F-format string=w152:string)  [unwired: 2 in]
                                n996 = case shown="真" w178 {
                                tunnel: ["1" "0"] -> w153
                                frame False {
                                }
                                frame True {
                                }
                                }
                                n997 = local read "Analog_back"() -> (w182:string[][])
                                n998 = call "误差计算.vi"("第几组"=w159, "选择?"=w166, "允许误差"=w173, "模拟量量程范围"=w167, "设定值_1"=w174, "反馈值_1"=w155) -> ("误差_1"=w163:dbl, "合格_1?"=w157:bool)  [unwired: 3 in, 1 out]
                                n999 = Number To Fractional String(number=w163, precision (6)=i16 3 ("精度(6)")) -> (F-format string=w162:string)  [unwired: 2 in]
                                n1000 = Replace Array Subset(array=w182, new element #1=w153, index (row) #1=w156, index (col) #1=0 ("y"), new element #2=w152, index (row) #2=w156, index (col) #2=1 ("y"), new element #3=w162, index (row) #3=w156, index (col) #3=2 ("y")) -> (w181:string[][])
                                n1001 = local read "合格？"() -> (w161:bool[][])
                                n1002 = local write "Analog_back"(w181) -> ()
                                n1003 = disable-structure shown="禁用" {
                                disable-tunnel: w156 -> [w185 _]
                                disable-tunnel: w153 -> [w184 _]
                                disable-tunnel: w152 -> [w183 _]
                                frame Disabled {
                                n1004 = Format Into String(format string="第组%d,,跳变值%s,发送值%s", w185, w184, w183) -> (resulting string=w187:string)  [unwired: 2 in, 1 out]
                                n1005 = call "显示对话框信息3"("Message"=w187) -> ()  [unwired: 9 in, 2 out]
                                }
                                frame Enabled {
                                }
                                }
                                n1006 = Replace Array Subset(array=w161, new element=w157, index (row)=w159, index (col)=0 ("禁用的索引 (列)")) -> (w160:bool[][])
                                n1007 = local write "合格？"(w160) -> ()
                              }
                              frame 2 {
                                n1008 = local read "第几组数据"() -> (w192:i32)
                                n1009 = global read "试验配置信息.vi" "允许误差"() -> (w211:dbl[])
                                n1010 = global read "试验配置信息.vi" "参数A1"() -> (w210:dbl[])
                                n1011 = global read "试验配置信息.vi" "Max"() -> (w206:dbl[])
                                n1012 = global read "试验配置信息.vi" "min"() -> (w205:dbl[])
                                n1013 = local read "发送值"() -> (w209:dbl)
                                n1014 = local read "最近一次跳变防线值"() -> (w215:i32)
                                n1015 = Index Array(array=w210, index=w192) -> (element=w208:dbl)
                                n1016 = Index Array(array=w206, index=w192) -> (element=w203:dbl)
                                n1017 = Index Array(array=w205, index=w192) -> (element=w202:dbl)
                                n1018 = Index Array(array=w211, index=w192) -> (element=w207:dbl)
                                n1019 = Subtract(x=w203, y=w202) -> (x-y=w204:dbl)
                                n1020 = Absolute Value(x=w204) -> (abs(x)=w201:dbl)
                                n1021 = local read "数组_选择"() -> (w200:bool[])
                                n1022 = local read "第几组数据"() -> (w199:i32)
                                n1023 = Equal To 0?(x=w215) -> (x = 0?=w216:bool)
                                n1024 = Number To Fractional String(number=w209, precision (6)=i16 3 ("精度(6)")) -> (F-format string=w212:string)  [unwired: 2 in]
                                n1025 = case shown="假" w216 {
                                tunnel: ["1" "0"] -> w214
                                frame False {
                                }
                                frame True {
                                }
                                }
                                n1026 = local read "Analog_back"() -> (w220:string[][])
                                n1027 = call "误差计算.vi"("第几组"=w192, "选择?"=w200, "允许误差"=w207, "模拟量量程范围"=w201, "设定值_1"=w208, "反馈值_1"=w209) -> ("误差_1"=w196:dbl, "合格_1?"=w190:bool)  [unwired: 3 in, 1 out]
                                n1028 = Number To Fractional String(number=w196, precision (6)=i16 3 ("精度(6)")) -> (F-format string=w195:string)  [unwired: 2 in]
                                n1029 = Replace Array Subset(array=w220, new element #1=w214, index (row) #1=w199, index (col) #1=3 ("y"), new element #2=w212, index (row) #2=w199, index (col) #2=4 ("y"), new element #3=w195, index (row) #3=w199, index (col) #3=5 ("y")) -> (w219:string[][])
                                n1030 = local read "合格？"() -> (w194:bool[][])
                                n1031 = local write "Analog_back"(w219) -> ()
                                n1032 = Replace Array Subset(array=w194, new element=w190, index (row)=w192, index (col)=1 ("禁用的索引 (列)")) -> (w193:bool[][])
                                n1033 = local write "合格？"(w193) -> ()
                              }
                              frame 3 {
                                n1034 = local read "第几组数据"() -> (w225:i32)
                                n1035 = local read "合格？"() -> (w227:bool[][])
                                n1036 = Replace Array Subset(array=w227, new element=FALSE, index (row)=w225, index (col)=0) -> (w226:bool[][])
                                n1037 = local write "合格？"(w226) -> ()
                              }
                            }
                          }
                        }
                      }
                    }
                  }
                  frame True {
                    # "收到第一个反馈值 记录首次跳变方向"
                    n1038 = local read "反馈值"() -> (w228:i32)
                    n1039 = local write "最近一次跳变防线值"(w228) -> ()
                  }
                }
              }
              frame #2 {
                n1040 = local read "第几组数据"() -> (w230:i32)
                n1041 = local read "合格？"() -> (w234:bool[][])
                n1042 = Index Array(array=w234, index (row)=w230) -> (element=w235:bool[])  [unwired: 1 in]
                n1043 = And Array Elements(Boolean array=w235) -> (logical AND=w232:bool)
                n1044 = local read "数组_选择"() -> (w231:bool[])
                n1045 = Index Array(array=w231, index=w230) -> (element=w233:bool)
                n1046 = case shown="真" w233 {
                  tunnel: [cluster{u32, u32}[] [{12369084, 12369084}] w270] -> w229
                  tunnel: w232 -> [_ w269]
                  frame False {
                  }
                  frame True {
                    n1047 = case shown="真" w269 {
                      tunnel: [cluster{u32, u32}[] [{16730410, 16711680}] cluster{u32, u32}[] [{61205, 6618880}]] -> w270
                      frame False {
                      }
                      frame True {
                      }
                    }
                  }
                }
                n1048 = case shown="31" w230 {
                  tunnel: w229 -> [w236 w237 w238 w239 w240 w241 w242 w243 w244 w245 w246 w247 w248 w249 w250 w251 w252 w253 w254 w255 w256 w257 w258 w259 w260 w261 w262 w263 w264 w265 w266 w267]
                  frame 0, Default {
                    n1049 = property on="light_1" class="Bool (严格)"("Colors [4]"=w236) -> ()  [unwired: 2 in, 2 out]
                  }
                  frame 1 {
                    n1050 = property on="light_2" class="Bool (严格)"("Colors [4]"=w237) -> ()  [unwired: 2 in, 2 out]
                  }
                  frame 2 {
                    n1051 = property on="light_3" class="Bool (严格)"("Colors [4]"=w238) -> ()  [unwired: 2 in, 2 out]
                  }
                  frame 3 {
                    n1052 = property on="light_4" class="Bool (严格)"("Colors [4]"=w239) -> ()  [unwired: 2 in, 2 out]
                  }
                  frame 4 {
                    n1053 = property on="light_5" class="Bool (严格)"("Colors [4]"=w240) -> ()  [unwired: 2 in, 2 out]
                  }
                  frame 5 {
                    n1054 = property on="light_6" class="Bool (严格)"("Colors [4]"=w241) -> ()  [unwired: 2 in, 2 out]
                  }
                  frame 6 {
                    n1055 = property on="light_7" class="Bool (严格)"("Colors [4]"=w242) -> ()  [unwired: 2 in, 2 out]
                  }
                  frame 7 {
                    n1056 = property on="light_8" class="Bool (严格)"("Colors [4]"=w243) -> ()  [unwired: 2 in, 2 out]
                  }
                  frame 8 {
                    n1057 = property on="light_9" class="Bool (严格)"("Colors [4]"=w244) -> ()  [unwired: 2 in, 2 out]
                  }
                  frame 9 {
                    n1058 = property on="light_10" class="Bool (严格)"("Colors [4]"=w245) -> ()  [unwired: 2 in, 2 out]
                  }
                  frame 10 {
                    n1059 = property on="light_11" class="Bool (严格)"("Colors [4]"=w246) -> ()  [unwired: 2 in, 2 out]
                  }
                  frame 11 {
                    n1060 = property on="light_12" class="Bool (严格)"("Colors [4]"=w247) -> ()  [unwired: 2 in, 2 out]
                  }
                  frame 12 {
                    n1061 = property on="light_13" class="Bool (严格)"("Colors [4]"=w248) -> ()  [unwired: 2 in, 2 out]
                  }
                  frame 13 {
                    n1062 = property on="light_14" class="Bool (严格)"("Colors [4]"=w249) -> ()  [unwired: 2 in, 2 out]
                  }
                  frame 14 {
                    n1063 = property on="light_15" class="Bool (严格)"("Colors [4]"=w250) -> ()  [unwired: 2 in, 2 out]
                  }
                  frame 15 {
                    n1064 = property on="light_16" class="Bool (严格)"("Colors [4]"=w251) -> ()  [unwired: 2 in, 2 out]
                  }
                  frame 16 {
                    n1065 = property on="light_17" class="Bool (严格)"("Colors [4]"=w252) -> ()  [unwired: 2 in, 2 out]
                  }
                  frame 17 {
                    n1066 = property on="light_18" class="Bool (严格)"("Colors [4]"=w253) -> ()  [unwired: 2 in, 2 out]
                  }
                  frame 18 {
                    n1067 = property on="light_19" class="Bool (严格)"("Colors [4]"=w254) -> ()  [unwired: 2 in, 2 out]
                  }
                  frame 19 {
                    n1068 = property on="light_20" class="Bool (严格)"("Colors [4]"=w255) -> ()  [unwired: 2 in, 2 out]
                  }
                  frame 20 {
                    n1069 = property on="light_21" class="Bool (严格)"("Colors [4]"=w256) -> ()  [unwired: 2 in, 2 out]
                  }
                  frame 21 {
                    n1070 = property on="light_22" class="Bool (严格)"("Colors [4]"=w257) -> ()  [unwired: 2 in, 2 out]
                  }
                  frame 22 {
                    n1071 = property on="light_23" class="Bool (严格)"("Colors [4]"=w258) -> ()  [unwired: 2 in, 2 out]
                  }
                  frame 23 {
                    n1072 = property on="light_24" class="Bool (严格)"("Colors [4]"=w259) -> ()  [unwired: 2 in, 2 out]
                  }
                  frame 24 {
                    n1073 = property on="light_25" class="Bool (严格)"("Colors [4]"=w260) -> ()  [unwired: 2 in, 2 out]
                  }
                  frame 25 {
                    n1074 = property on="light_26" class="Bool (严格)"("Colors [4]"=w261) -> ()  [unwired: 2 in, 2 out]
                  }
                  frame 26 {
                    n1075 = property on="light_27" class="Bool (严格)"("Colors [4]"=w262) -> ()  [unwired: 2 in, 2 out]
                  }
                  frame 27 {
                    n1076 = property on="light_28" class="Bool (严格)"("Colors [4]"=w263) -> ()  [unwired: 2 in, 2 out]
                  }
                  frame 28 {
                    n1077 = property on="light_29" class="Bool (严格)"("Colors [4]"=w264) -> ()  [unwired: 2 in, 2 out]
                  }
                  frame 29 {
                    n1078 = property on="light_30" class="Bool (严格)"("Colors [4]"=w265) -> ()  [unwired: 2 in, 2 out]
                  }
                  frame 30 {
                    n1079 = property on="light_31" class="Bool (严格)"("Colors [4]"=w266) -> ()  [unwired: 2 in, 2 out]
                  }
                  frame 31 {
                    n1080 = property on="light_32" class="Bool (严格)"("Colors [4]"=w267) -> ()  [unwired: 2 in, 2 out]
                  }
                }
              }
              frame #3 {
                n1081 = local write "bRecv"(TRUE) -> ()
              }
            }
          }
        }
        n1082 = local read "退出？"() -> (w128:bool)
      }
      n1083 = Release Notifier(notifier=w116) -> ()  [unwired: 2 in, 3 out]
    }
  }
  n1084 = disable-structure shown="启用" {
    frame Enabled {
      n1085 = for {
        N: 32 -> [_]
        i -> [w547]
        n1086 = for {
          N: 6 -> [_]
          tunnel: w547 -> [w550]
          i -> [w551]
          n1087 = Bundle(w550, w551) -> (w554:cluster{i32, i32})  [unwired: 1 in]
          n1088 = property on="Analog_back" class="Tbl (严格)"("Active Cell"=w554) -> (error out=w552:errorcluster)  [unwired: 2 in, 1 out]
          n1089 = property on="Analog_back" class="Tbl (严格)"(error in=w552, "Justify"=enum16{"Left", "Center", "Right"}."Center" ("活动单元格:单元格对齐")) -> ()  [unwired: 1 in, 2 out]
        }
        n1090 = Wait Until Next ms Multiple(millisecond multiple=u32 10 ("毫秒倍数")) -> ()  [unwired: 1 out]
      }
    }
    frame Disabled {
    }
  }
